vi "NEW数据采集传输系统.vi"() -> ()   [LabVIEW 2016, in "数据传输系统.lvlib"]
uses:
  <vilib>/Averna/Notify Icon/NotifyIcon.llb/BalloonIcon.ctl
  <vilib>/Utility/miscctls.llb/LVPointTypeDef.ctl
  <vilib>/Utility/config.llb/Read Key (String).vi
  <vilib>/Averna/Notify Icon/NotifyIcon.llb/GetSelectedItemEvent.vi
  <vilib>/Averna/Notify Icon/NotifyIcon.llb/SetVisible.vi
  <vilib>/Averna/Notify Icon/NotifyIcon.llb/SetMenuDefaultItem.vi
  <vilib>/Averna/Notify Icon/NotifyIcon.llb/SetTipText.vi
  <vilib>/Utility/config.llb/NI_LVConfig.lvlib
  data/FreeMem.dll
  <vilib>/Averna/Notify Icon/NotifyIcon.llb/NotifyIcon.lvclass
panel:
  out "错误输出":errorcluster
  in  "停止输入":bool caption="停止 2"
  in  "系统编码选择框":string(combo)="地表水质量监测"
  in  "数据发送通道":enum16{"TCP", "VISA"}(ring)
  in  "baud rate":u32=9600 caption="波特率"
  in  "VISA resource name":refnum<visa-resource-name> caption="VISA资源名称"
  in  "实时数据发送时间间隔/min":i32=1
  in  "数据组合发送":bool
  in  "日志、参数发送":bool
  in  "2011发送":bool
  in  "判断数据反馈":bool
  in  "数据发送协议":enum16{"2005-212协议", "2017-212协议"}(ring)=enum."2017-212协议"
  in  "重发时间":T1(ring)
  in  "重发日期":T2(ring)
  in  "开机启动":bool
  in  "确定更改起始时间":bool
  in  "更改起始时间":bool
  in  "数据发送起始时间":timestamp format="%<%.3X\n%Y/%m/%d>T"
  in  "每周自动重发":bool=TRUE
  in  "确定":bool
  in  "返回":bool
  in  "PW":string
  in  "MN":string
  in  "PORT":string
  in  "IP":string
  in  "站点设备":string
  in  "站点名称":string
  out "设置超时时间/min":i32=1
  out "状态信息":T3={"1st Error to Convert "=63, "步骤 "=enum."发送数据", "元素"="实时数据", "TCP服务端掉线计数"=0, "TCP掉线时间节点"="2019/05/08 15:24:17"} {"1st Error to Convert" items=["无错误", "参数错误", "内存已满", "超出区域", "文件结束", "文件已打开", "一般文件IO错误", "未找到文件", "文件权限错误", "磁盘已满", "路径副本", "打开过多文件", "未启用", "未找到资源文件", "无法添加资源", "未找到资源", "未找到图像", "图像内存错误", "画笔不存在", "配置错误类型", "配置未找到解析段", "配置解析错误", "配置内存错误", "错误外部代码格式", "错误外部代码偏移量", "外部代码不存在", "空窗口", "销毁窗口错误", "空菜单", "打印已中止", "错误打印记录", "打印驱动程序错误", "打印时窗口错误", "打印时内存错误", "打印对话框错误", "一般打印错误", "无效设备引用句柄", "设备未找到", "设备参数错误", "设备单位错误", "无法打开设备", "设备调用已中止", "一般错误", "用户已取消", "对象ID过低", "对象ID过高", "对象不在堆中", "未知的堆", "错误DefProc ID", "DefProc不在表格中", "范围外信息", "空方法", "未知信息", "不支持管理器调用", "错误地址", "连接过程中", "连接超时", "连接过程中", "不支持网络属性", "网络错误", "正在使用的地址", "系统缺少内存", "连接已中止", "连接已拒绝", "连接未建立", "连接已建立", "连接已关闭", "初始化错误（交互应用程序管理器）", "错误事件发生", "等待无约束事件发生处理程序", "事件发生队列溢出", "错误路径", "未发出信号量", "未识别类型（交互应用程序管理器）"]}
  out "数据接收超时指示灯":bool
  out "空闲时间/s":string
  out "系统时间":string
  out "实时小时数据上传":bool
  out "系统状态改变":bool
  out "软件版本":string
  out "掉线指示":bool
  out "核查数据上传":bool
  out "配置信息":T4
  in  "参数配置":bool
  out "反控数据发送":bool
  out "读取报文显示":string
  out "发送报文显示":string
  out "心跳包":bool
  out "通信状态":bool
  # "数 据 采 集 传 输 系 统"
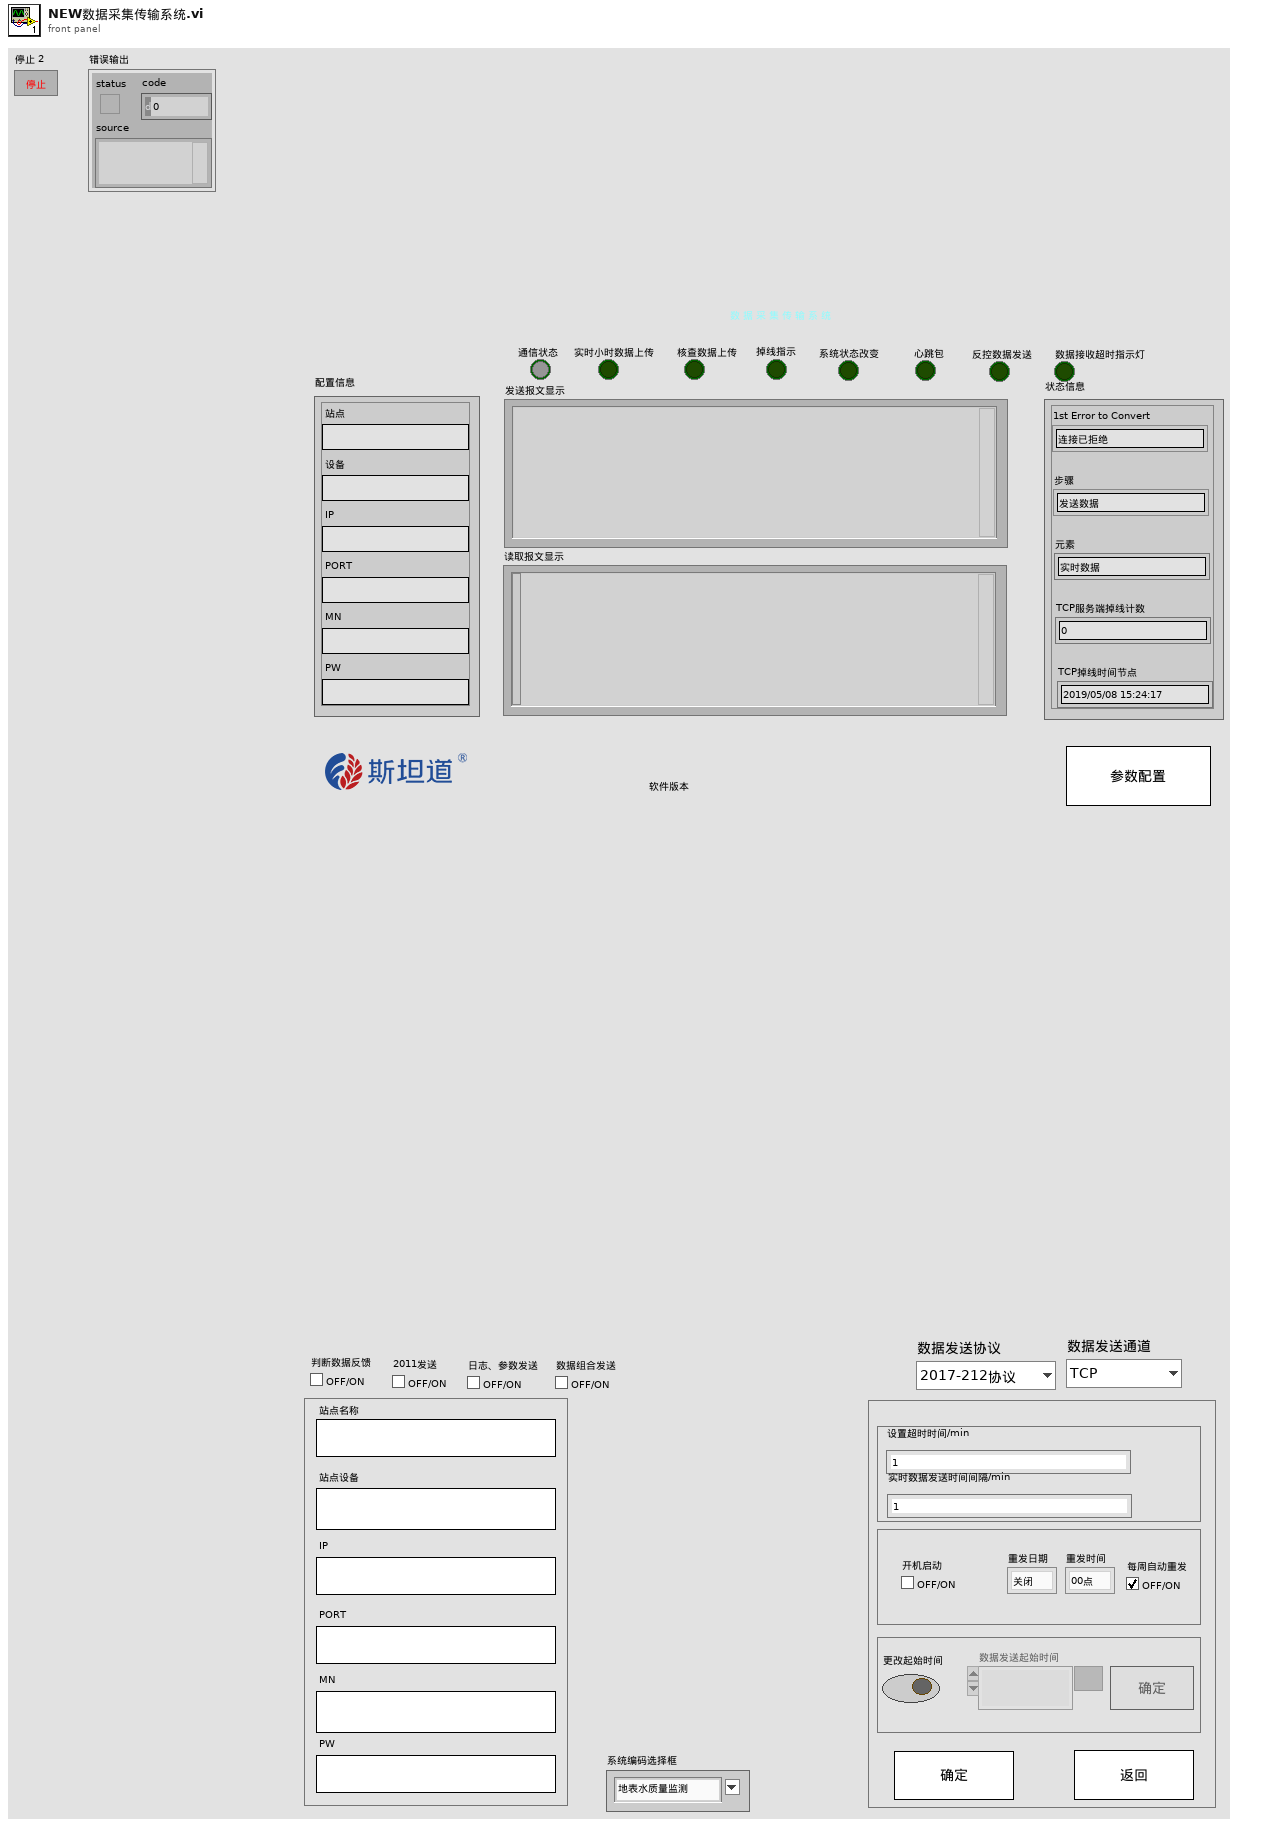
[diagram p1: front panel]
types:
  T1 = enum16{"00点", "01点", "02点", "03点", "04点", "05点", "06点", "07点", "08点", "09点", "10点", "11点", "12点", "13点", "14点", "15点", "16点", "17点", "18点", "19点", "20点", "21点", "22点", "23点"}
  T2 = enum16{"关闭", "星期日", "星期一", "星期二", "星期三", "星期四", "星期五", "星期六"}
  T3 = cluster{"1st Error to Convert ":i32, "步骤 ":enum16{"打开连接", "发送数据", "读取数据", "数据处理", "关闭连接"}, "元素":string, "TCP服务端掉线计数":i32, "TCP掉线时间节点":string}
  T4 = cluster{"站点":string, "设备":string, "IP":string, "PORT":string, "MN":string, "PW":string}
  T5 = typedef "LVPointTypeDef.ctl" = cluster{"Horizontal":i16, "Vertical":i16}
  T6 = cluster{"CODMn":bool, "CODCr":bool, "DO":bool, "铜":bool, "PH":bool, "氨氮":bool, "比电导率":bool, "水温":bool, "盐度(海水)":bool, "浊度":bool, "总氮":bool, "总磷":bool, "叶绿素a":bool, "藻密度":bool, "水位":bool, "流速":bool, "瞬时流量":bool, "累积流量":bool}
  T7 = typedef "NI_LVConfig.lvlib/Config Data RefNum.ctl" = refnum<k1>
  T8 = typedef "LVDateTimeRec.ctl" = cluster{"秒数的小数部分":dbl, "秒":i32, "分":i32, "时":i32, "日":i32, "月":i32, "年":i32, "天数（周）":i32, "天数（年）":i32, "DST":i32}
  T9 = typedef "imagedata.ctl" = cluster{"image type":i32, "image depth":i32, "image":u8[], "mask":u8[], "colors":u32[], "Rectangle":cluster{"left":i16, "top":i16, "right":i16, "bottom":i16}}
  T10 = enum8{"Enabled", "Disabled", "Disabled and Grayed Out"}
  T11 = enum32{"invalid app kind", "Development System", "Run Time System", "Student Edition", "Embedded LabVIEW", "Evaluation", "Custom"}
  T12 = enum32{"Invalid", "Standard", "Closed", "Hidden", "Minimized", "Maximized"}
  T13 = typedef "NotifyIcon.lvlib/NotifyIcon.lvclass/BalloonIcon.ctl" = enum32{"None", "Information", "Warning", "Error"}
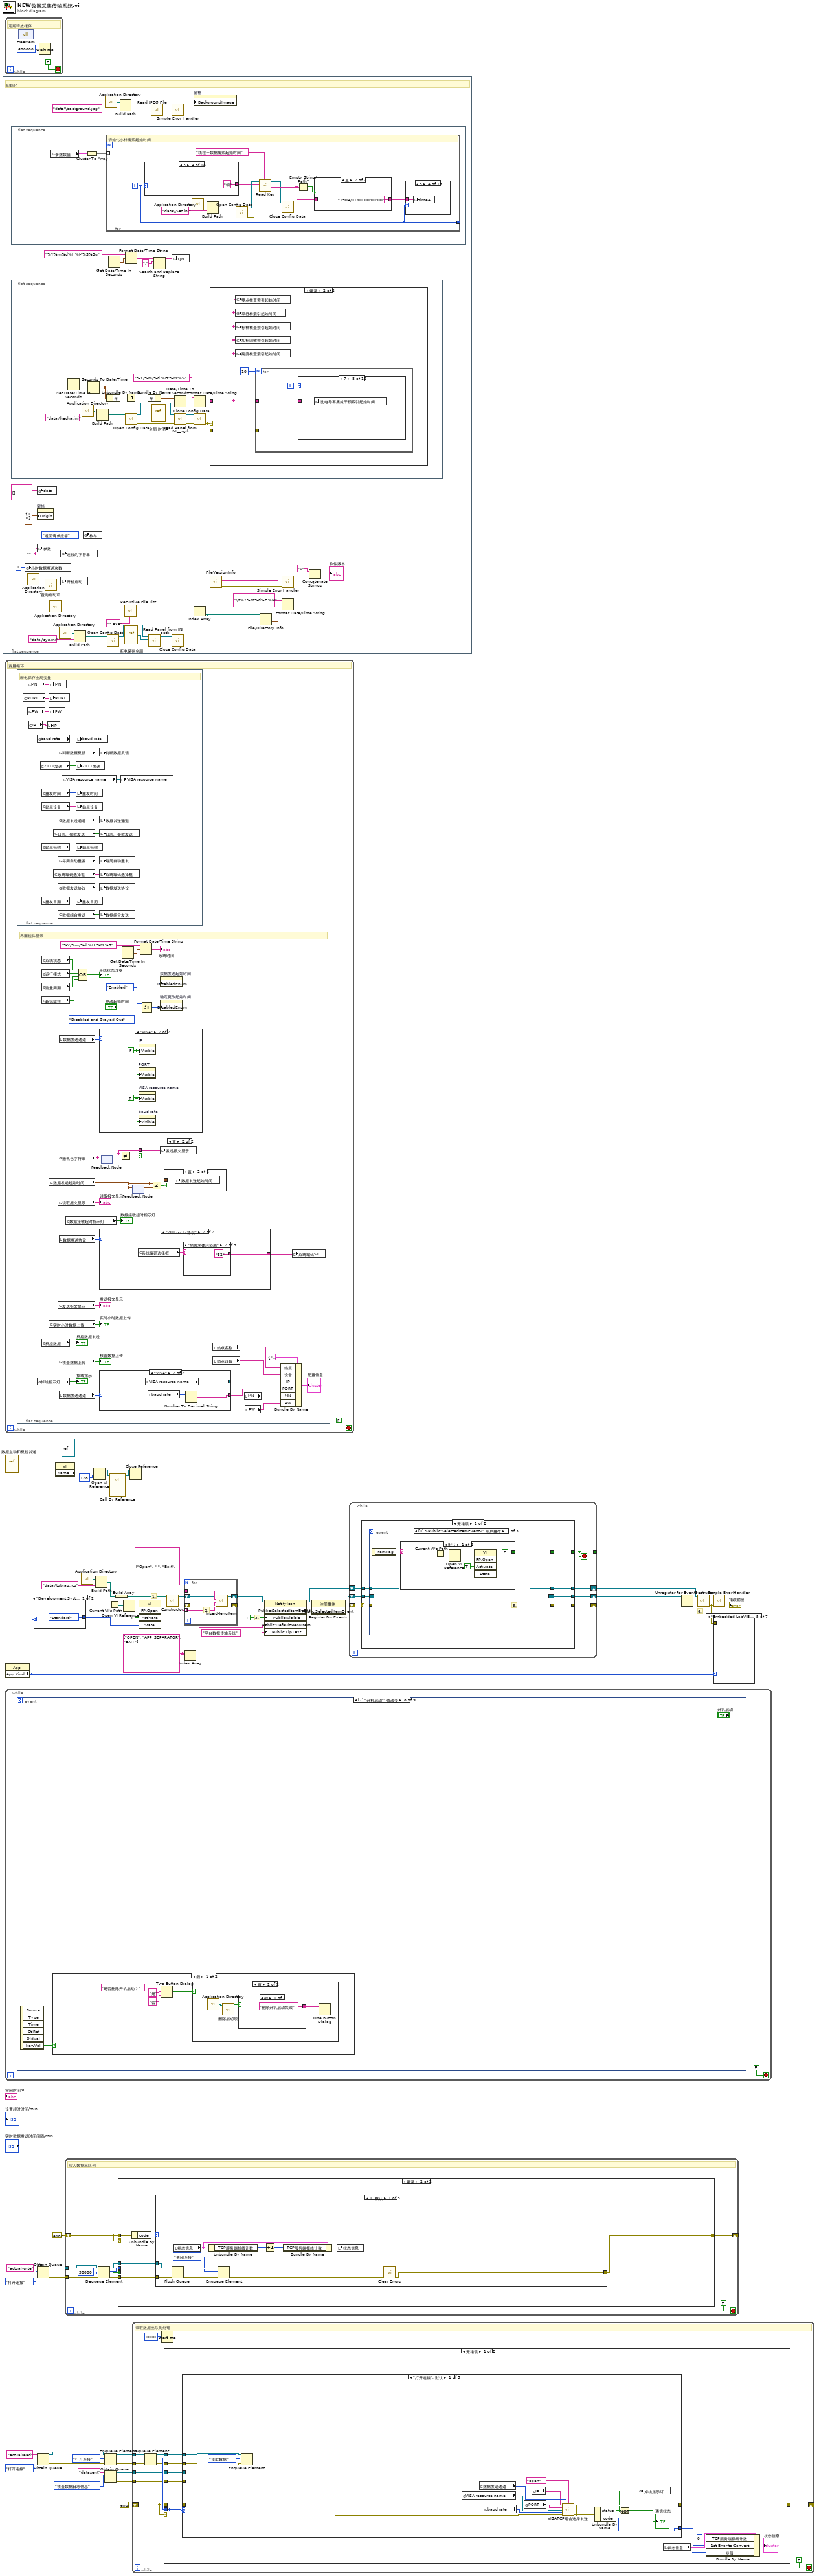
[diagram p0: block diagram]
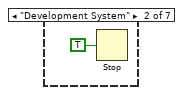
[diagram p3: hidden frame]
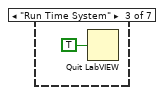
[diagram p4: hidden frame]
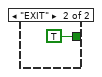
[diagram p8: hidden frame]
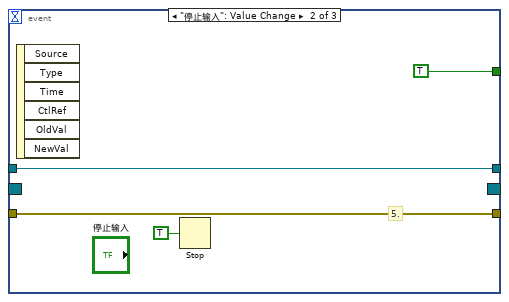
[diagram p9: hidden frame]
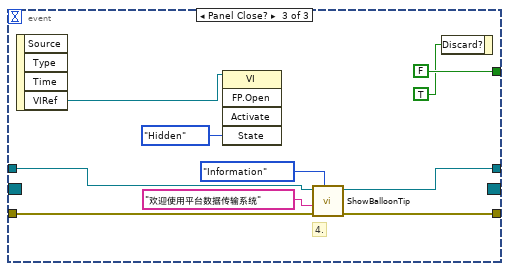
[diagram p10: hidden frame]
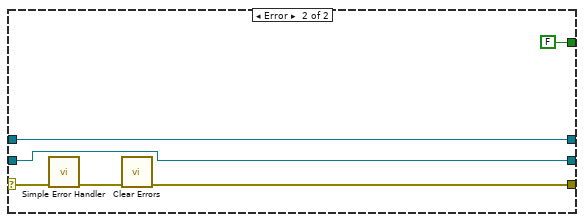
[diagram p11: hidden frame]
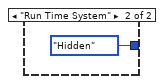
[diagram p12: hidden frame]
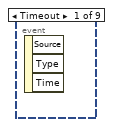
[diagram p13: hidden frame]
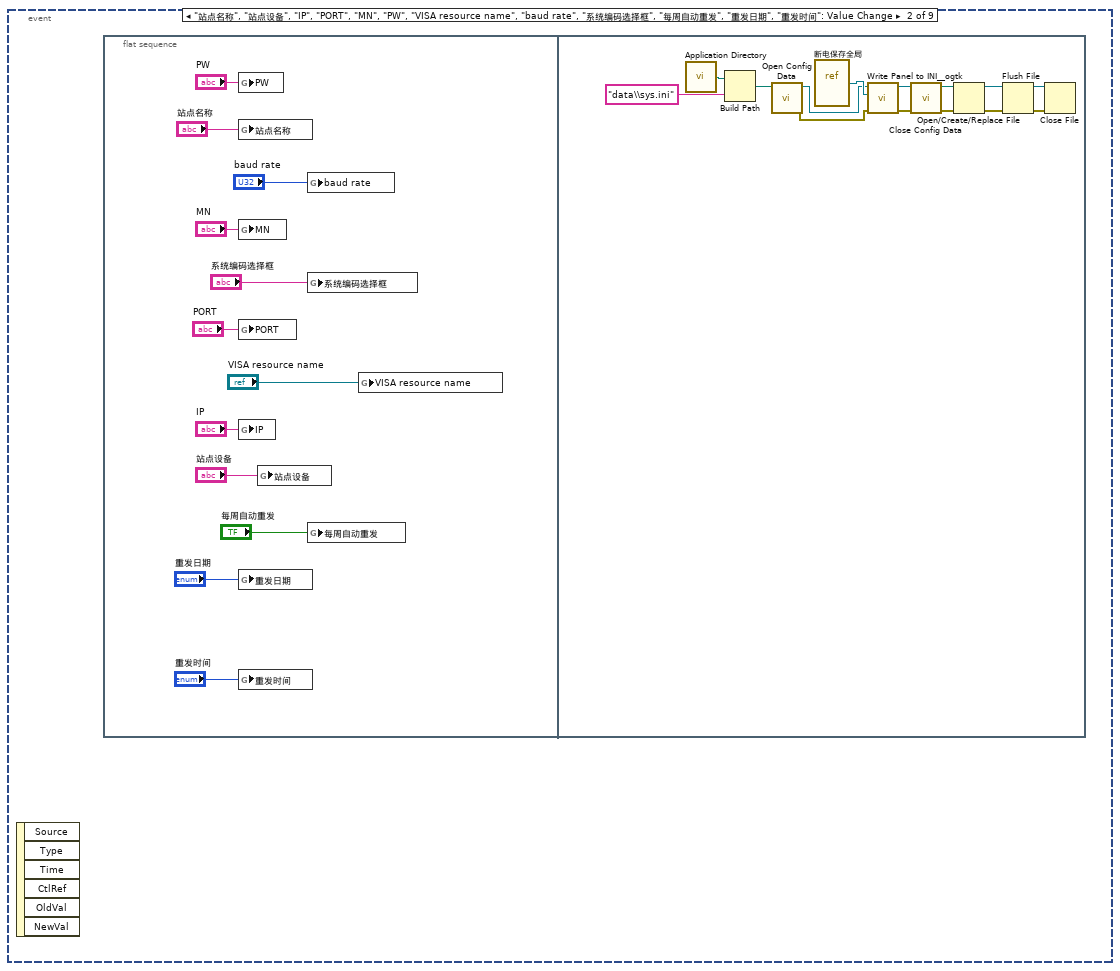
[diagram p14: hidden frame]
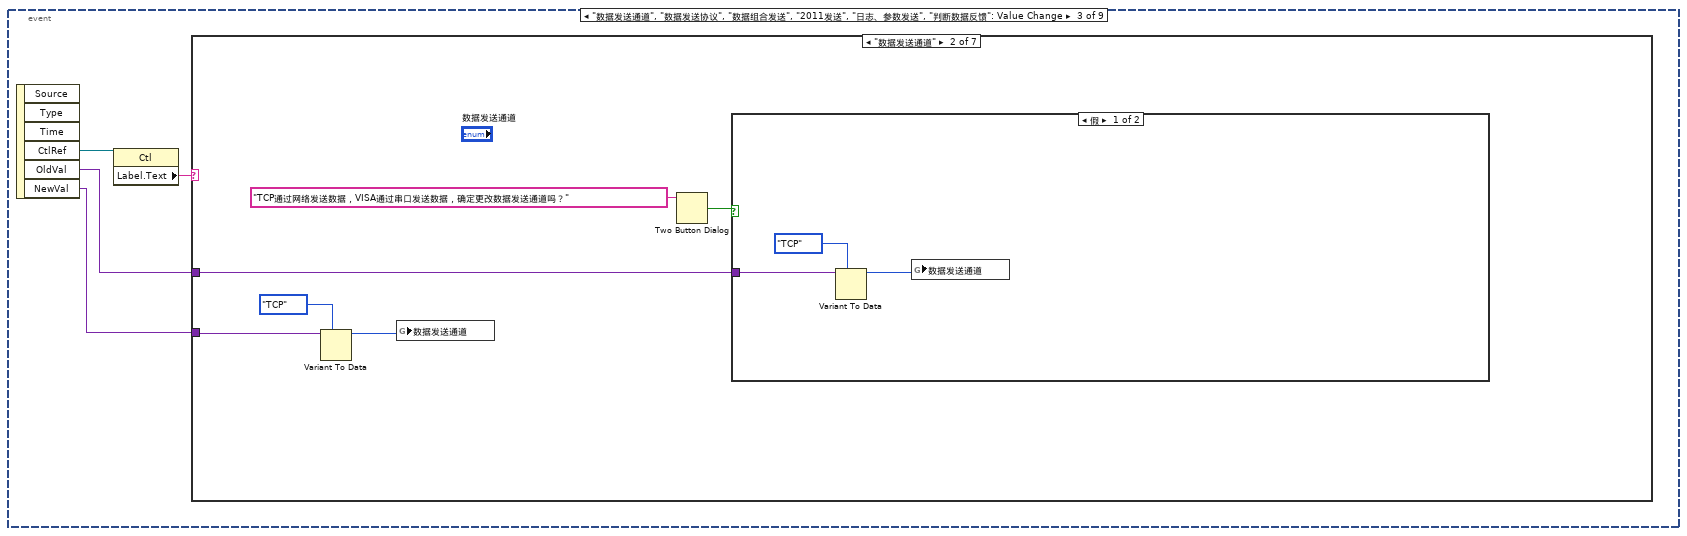
[diagram p15: hidden frame]
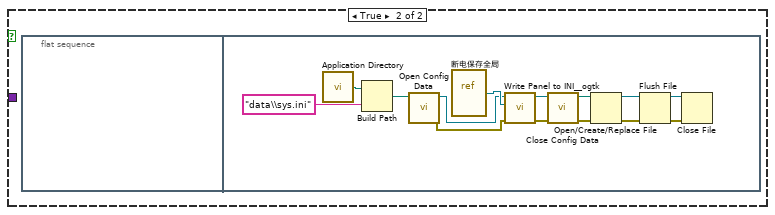
[diagram p17: hidden frame]
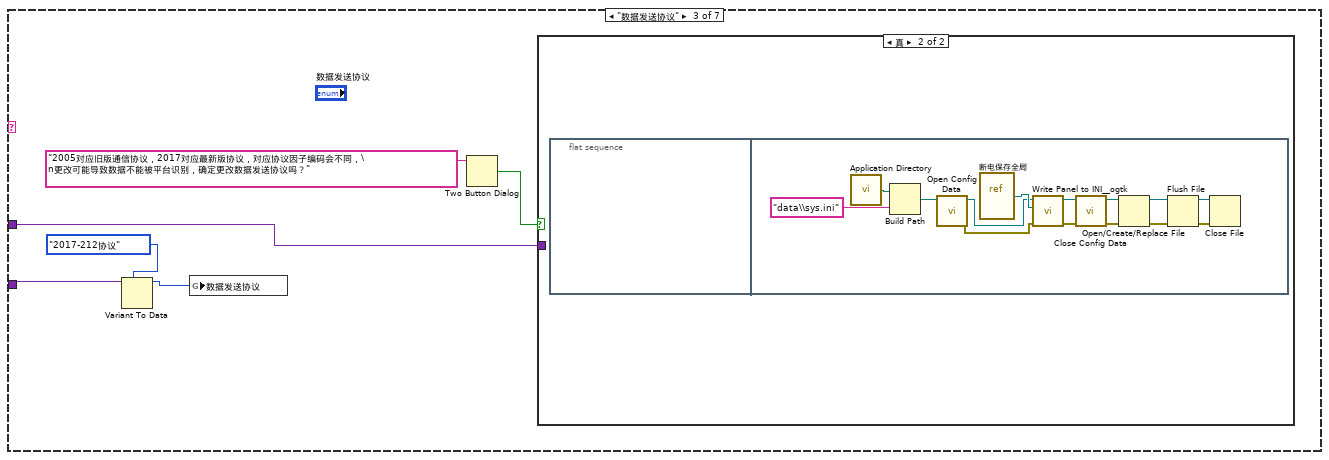
[diagram p18: hidden frame]
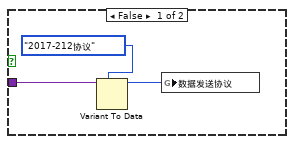
[diagram p19: hidden frame]
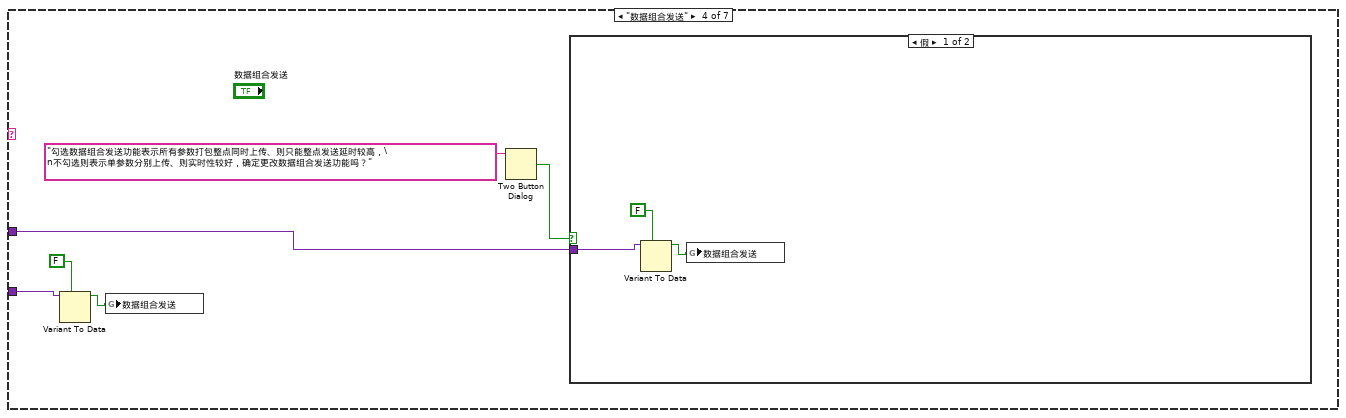
[diagram p20: hidden frame]
diagram:
  w13 = string[] ["OPEN", "APP_SEPARATOR", "EXIT"]
  # "6."
  # "3."
  # "1."
  n1 = flat-sequence {
    frame #0 {
      w89 = "" ("参数")
      # "初始化"
      n2 = flat-sequence {
        frame #0 {
          n3 = global read "全局1.vi" "参数数值"() -> (w92:T6)
          n4 = Cluster To Array(cluster=w92) -> (array=w93:bool[])
          n5 = for {
            tunnel: w93 -> [_] mode=indexing
            tunnel: [w96] -> _
            i -> [w96]
            # "初始化水样搜索起始时间"
            n6 = case shown="3" w96 {
              tunnel: ["CODMn" "CODCr" "DO" "铜" "PH" "氨氮" "比电导率" "水温" "盐度(海水)" "浊度" "总氮" "总磷" "叶绿素a" "藻密度" "水位" "流速" "瞬时流量" "累积流量"] -> w100
              frame 0, Default {
              }
              frame 1 {
              }
              frame 2 {
              }
              frame 3 {
              }
              frame 4 {
              }
              frame 5 {
              }
              frame 6 {
              }
              frame 7 {
              }
              frame 8 {
              }
              frame 9 {
              }
              frame 10 {
              }
              frame 11 {
              }
              frame 12 {
              }
              frame 13 {
              }
              frame 14 {
              }
              frame 15 {
              }
              frame 16 {
              }
              frame 17 {
              }
            }
            n7 = call <vilib>:"Application Directory.vi"() -> ("Application Directory"=w106:path)
            n8 = Build Path(base path=w106, name or relative path="data\\Set.ini" ("名称或相对路径")) -> (appended path=w104:path)
            n9 = call <vilib>:"Open Config Data.vi"("configuration file path"=w104) -> ("error out"=w102:errorcluster, "refnum"=w103:T7)  [unwired: 8 in, 1 out]
            n10 = call-poly <vilib>:"Read Key.vi"("section"="线程一数据搜索起始时间", "error in (no error)"=w102, "key"=w100, "refnum"=w103) -> ("error out"=w94:errorcluster, "value"=w97:string, "refnum out"=w95:T7)  [unwired: 4 in, 1 out]
            n11 = call <vilib>:"Close Config Data.vi"("error in (no error)"=w94, "refnum"=w95) -> ()  [unwired: 8 in, 2 out]
            n12 = Empty String/Path?(string/path=w97) -> (empty?=w99:bool)
            n13 = case shown="真" w99 {
              tunnel: [w107 "1904/01/01 00:00:00"] -> w98
              tunnel: w97 -> [w107 _]
              frame False {
              }
              frame True {
              }
            }
            n14 = case shown="3" w96 {
              tunnel: w98 -> [w109 w110 w111 w112 w113 w114 w115 w116 w117 w118 w119 w120 w121 w122 w123 w124 w125 w126]
              frame 0, Default {
                n15 = global write "全局 水样时间.vi" "time1"(w109) -> ()
              }
              frame 1 {
                n16 = global write "全局 水样时间.vi" "time2"(w110) -> ()
              }
              frame 2 {
                n17 = global write "全局 水样时间.vi" "time3"(w111) -> ()
              }
              frame 3 {
                n18 = global write "全局 水样时间.vi" "time4"(w112) -> ()
              }
              frame 4 {
                n19 = global write "全局 水样时间.vi" "time5"(w113) -> ()
              }
              frame 5 {
                n20 = global write "全局 水样时间.vi" "time6"(w114) -> ()
              }
              frame 6 {
                n21 = global write "全局 水样时间.vi" "time7"(w115) -> ()
              }
              frame 7 {
                n22 = global write "全局 水样时间.vi" "time8"(w116) -> ()
              }
              frame 8 {
                n23 = global write "全局 水样时间.vi" "time9"(w117) -> ()
              }
              frame 9 {
                n24 = global write "全局 水样时间.vi" "time10"(w118) -> ()
              }
              frame 10 {
                n25 = global write "全局 水样时间.vi" "time11"(w119) -> ()
              }
              frame 11 {
                n26 = global write "全局 水样时间.vi" "time12"(w120) -> ()
              }
              frame 12 {
                n27 = global write "全局 水样时间.vi" "time13"(w121) -> ()
              }
              frame 13 {
                n28 = global write "全局 水样时间.vi" "time14"(w122) -> ()
              }
              frame 14 {
                n29 = global write "全局 水样时间.vi" "time15"(w123) -> ()
              }
              frame 15 {
                n30 = global write "全局 水样时间.vi" "time16"(w124) -> ()
              }
              frame 16 {
                n31 = global write "全局 水样时间.vi" "time17"(w125) -> ()
              }
              frame 17 {
                n32 = global write "全局 水样时间.vi" "time18"(w126) -> ()
              }
            }
          }
        }
      }
      n33 = flat-sequence {
        frame #0 {
          n34 = Get Date/Time In Seconds() -> (seconds since 1Jan1904=w161:timestamp)
          n35 = call <vilib>:"Application Directory.vi"() -> ("Application Directory"=w151:path)
          n36 = Seconds To Date/Time(time stamp (now)=w161) -> (date time rec=w159:T8)  [unwired: 1 in]
          n37 = Build Path(base path=w151, name or relative path="data\\hecha.ini" ("名称或相对路径")) -> (appended path=w153:path)
          n38 = Unbundle By Name(w159) -> ("年"=w160:i32)
          n39 = Decrement(x=w160) -> (x-1=w158:i32)
          n40 = call <vilib>:"Open Config Data.vi"("configuration file path"=w153) -> ("error out"=w147:errorcluster, "refnum"=w148:T7)  [unwired: 8 in, 1 out]
          n41 = Bundle By Name(cluster=w159, "年"=w158) -> (w156:T8)
          n42 = vi-ref "全局 时间2.vi"() -> (w149:refnum<vi>)
          n43 = Date/Time To Seconds(2:w156) -> (0:w157:timestamp)  [unwired: 1 in]
          n44 = call <userlib>:"Read Panel from INI__ogtk.vi"("error in (no error)"=w147, "VI ref"=w149, "refnum"=w148) -> ("error out"=w146:errorcluster, "refnum out"=w150:T7)  [unwired: 7 in]
          n45 = Format Date/Time String(time format string (%c)="%Y/%m/%d %H:%M:%S" ("时间格式字符串(%c)"), seconds (now)=w157) -> (date/time string=w154:string)  [unwired: 1 in]
          n46 = call <vilib>:"Close Config Data.vi"("error in (no error)"=w146, "refnum"=w150) -> ("error out"=w145:errorcluster)  [unwired: 8 in, 1 out]
          n47 = case shown="错误" w145 {
            tunnel: w154 -> [_ w164]
            tunnel: w145 -> [_ w163]
            frame No Error {
            }
            frame Error {
              n48 = global write "全局 时间2.vi" "零点核查索引起始时间"(w164) -> ()
              n49 = global write "全局 时间2.vi" "平行样索引起始时间"(w164) -> ()
              n50 = global write "全局 时间2.vi" "标样核查索引起始时间"(w164) -> ()
              n51 = global write "全局 时间2.vi" "加标回收索引起始时间"(w164) -> ()
              n52 = global write "全局 时间2.vi" "跨度核查索引起始时间"(w164) -> ()
              n53 = for {
                N: 10 -> [_]
                tunnel: w164 -> [w165]
                tunnel: w163 -> [_]
                i -> [w166]
                n54 = case shown="7" w166 {
                  tunnel: w165 -> [w167 w168 w169 w170 w171 w172 w173 w174 w175 w176]
                  frame 0, Default {
                    n55 = global write "全局 时间2.vi" "氨氮平行样索引起始时间"(w167) -> ()
                    n56 = global write "全局 时间2.vi" "氨氮零点核查索引起始时间"(w167) -> ()
                    n57 = global write "全局 时间2.vi" "氨氮集成干预索引起始时间"(w167) -> ()
                    n58 = global write "全局 时间2.vi" "氨氮跨度核查索引起始时间"(w167) -> ()
                  }
                  frame 1 {
                    n59 = global write "全局 时间2.vi" "总氮零点核查索引起始时间"(w168) -> ()
                    n60 = global write "全局 时间2.vi" "总氮平行样索引起始时间"(w168) -> ()
                    n61 = global write "全局 时间2.vi" "总氮跨度核查索引起始时间"(w168) -> ()
                    n62 = global write "全局 时间2.vi" "总氮集成干预索引起始时间"(w168) -> ()
                  }
                  frame 2 {
                    n63 = global write "全局 时间2.vi" "总磷零点核查索引起始时间"(w169) -> ()
                    n64 = global write "全局 时间2.vi" "总磷平行样索引起始时间"(w169) -> ()
                    n65 = global write "全局 时间2.vi" "总磷跨度核查索引起始时间"(w169) -> ()
                    n66 = global write "全局 时间2.vi" "总磷集成干预索引起始时间"(w169) -> ()
                  }
                  frame 3 {
                    n67 = global write "全局 时间2.vi" "CODMn零点核查索引起始时间"(w170) -> ()
                    n68 = global write "全局 时间2.vi" "CODMn平行样索引起始时间"(w170) -> ()
                    n69 = global write "全局 时间2.vi" "CODMn跨度核查索引起始时间"(w170) -> ()
                    n70 = global write "全局 时间2.vi" "CODMn集成干预索引起始时间"(w170) -> ()
                  }
                  frame 4 {
                    n71 = global write "全局 时间2.vi" "CODCr零点核查索引起始时间"(w171) -> ()
                    n72 = global write "全局 时间2.vi" "CODCr平行样索引起始时间"(w171) -> ()
                    n73 = global write "全局 时间2.vi" "CODCr跨度核查索引起始时间"(w171) -> ()
                    n74 = global write "全局 时间2.vi" "CODCr集成干预索引起始时间"(w171) -> ()
                  }
                  frame 5 {
                    n75 = global write "全局 时间2.vi" "DO集成干预索引起始时间"(w172) -> ()
                  }
                  frame 6 {
                    n76 = global write "全局 时间2.vi" "PH集成干预索引起始时间"(w173) -> ()
                  }
                  frame 7 {
                    n77 = global write "全局 时间2.vi" "比电导率集成干预索引起始时间"(w174) -> ()
                  }
                  frame 8 {
                    n78 = global write "全局 时间2.vi" "水温集成干预索引起始时间"(w175) -> ()
                  }
                  frame 9 {
                    n79 = global write "全局 时间2.vi" "浊度集成干预索引起始时间"(w176) -> ()
                  }
                }
              }
            }
          }
        }
      }
      n80 = global write "全局 小时数据发送次数.vi" "小时数据发送次数"(0 ("数值")) -> ()
      n81 = call <vilib>:"Application Directory.vi"() -> ("Application Directory"=w57:path)
      n82 = global write "全局 实时数据参数.vi" "data"(string[][] [] ("data")) -> ()
      n83 = property on="窗格" class="Pane"("Origin"=T5 {"Horizontal"=0, "Vertical"=0} ("原点")) -> ()  [unwired: 2 in, 2 out]
      n84 = global write "全局 实时数据参数.vi" "参数"(w89) -> ()
      n85 = call "查询启动项.vi"("启动文件路径"=w57) -> ("包含启动项"=w56:bool)  [unwired: 9 in, 1 out]
      n86 = call <vilib>:"Application Directory.vi"() -> ("Application Directory"=w68:path)
      n87 = call <vilib>:"Application Directory.vi"() -> ("Application Directory"=w61:path)
      n88 = global write "全局 实时数据参数.vi" "连接的字符串"(w89) -> ()
      n89 = local write "开机启动"(w56) -> ()
      n90 = Build Path(base path=w61, name or relative path="data\\sys.ini" ("名称或相对路径")) -> (appended path=w59:path)
      n91 = global write "全局1.vi" "枚举"(enum16{"返回请求应答", "上传数据", "返回执行结果"}."返回请求应答" ("枚举")) -> ()
      n92 = call <vilib>:"Application Directory.vi"() -> ("Application Directory"=w80:path)
      n93 = call <vilib>:"Open Config Data.vi"("configuration file path"=w59) -> ("error out"=w65:errorcluster, "refnum"=w64:T7)  [unwired: 8 in, 1 out]
      n94 = Get Date/Time In Seconds() -> (seconds since 1Jan1904=w85:timestamp)
      n95 = Build Path(base path=w80, name or relative path="data\\background.jpg" ("名称或相对路径")) -> (appended path=w79:path)
      n96 = call <vilib>:"Recursive File List.vi"("pattern"="*.exe", "Folder Path"=w68) -> ("All Files in Dir"=w75:path[])  [unwired: 5 in, 4 out]
      n97 = vi-ref "断电保存全局.vi"() -> (w63:refnum<vi>)
      n98 = Format Date/Time String(time format string (%c)="%Y%m%d%H%M%S%3u" ("时间格式字符串(%c)"), seconds (now)=w85) -> (date/time string=w84:string)  [unwired: 1 in]
      n99 = call <userlib>:"Read Panel from INI__ogtk.vi"("error in (no error)"=w65, "VI ref"=w63, "refnum"=w64) -> ("error out"=w58:errorcluster, "refnum out"=w62:T7)  [unwired: 7 in]
      n100 = call <vilib>:"Read JPEG File.vi"("path to JPEG file"=w79) -> ("error out"=w77:errorcluster, "image data"=w78:T9)  [unwired: 8 in, 1 out]
      n101 = Search and Replace String(input string=w84, search string="." ("搜索字符串")) -> (result string=w82:string)  [unwired: 6 in, 3 out]
      n102 = call <vilib>:"Simple Error Handler.vi"("error in (no error)"=w77) -> ()  [unwired: 4 in, 5 out]
      n103 = global write "全局1.vi" "QN"(w82) -> ()
      n104 = call <vilib>:"Close Config Data.vi"("error in (no error)"=w58, "refnum"=w62) -> ()  [unwired: 8 in, 2 out]
      n105 = property on="窗格" class="Pane"("BackgroundImage"=w78) -> ()  [unwired: 2 in, 2 out]
      n106 = Index Array(array=w75) -> (element=w74:path)  [unwired: 1 in]
      n107 = call <vilib>:"FileVersionInfo.vi"("Application Path in"=w74) -> ("error out"=w67:errorcluster, "File Version Info"=w70:string)  [unwired: 7 in, 2 out]
      n108 = File/Directory Info(path=w74) -> (last mod=w73:timestamp)  [unwired: 1 in, 6 out]
      n109 = call <vilib>:"Simple Error Handler.vi"("error in (no error)"=w67) -> ()  [unwired: 4 in, 5 out]
      n110 = Format Date/Time String(time format string (%c)="\n%Y%m%d%H%M" ("时间格式字符串(%c)"), seconds (now)=w73) -> (date/time string=w69:string)  [unwired: 1 in]
      n111 = Concatenate Strings("V" ("字符串"), w70, w69) -> (→"软件版本":string)
    }
  }
  n112 = while {
    stop <- FALSE stop-if-true
    # "定期释放缓存"
    n113 = dll-call lib="PTH2aabs F\tgitkrakenCC6平台数采程序 - V2.0.1（正式修改迭代版）dataFreeMem.dll" fn="FreeMem"() -> ()  [unwired: 4 in, 2 out]
    n114 = Wait (ms)(milliseconds to wait=u32 600000 ("等待时间（毫秒）")) -> ()  [unwired: 1 out]
  }
  n115 = while {
    stop <- FALSE stop-if-true
    # "变量循环"
    n116 = flat-sequence {
      frame #0 {
        # "断电保存全局变量"
        n117 = global read "断电保存全局.vi" "PORT"() -> (w248:string)
        n118 = global read "断电保存全局.vi" "MN"() -> (w247:string)
        n119 = global read "断电保存全局.vi" "PW"() -> (w246:string)
        n120 = global read "断电保存全局.vi" "IP"() -> (w249:string)
        n121 = global read "断电保存全局.vi" "baud rate"() -> (w244:u32)
        n122 = global read "断电保存全局.vi" "2011发送"() -> (w240:bool)
        n123 = global read "断电保存全局.vi" "重发时间"() -> (w234:T1)
        n124 = global read "断电保存全局.vi" "站点设备"() -> (w250:string)
        n125 = global read "断电保存全局.vi" "站点名称"() -> (w251:string)
        n126 = global read "断电保存全局.vi" "重发日期"() -> (w242:T2)
        n127 = local write "IP"(w249) -> ()
        n128 = local write "MN"(w247) -> ()
        n129 = local write "PORT"(w248) -> ()
        n130 = local write "PW"(w246) -> ()
        n131 = global read "断电保存全局.vi" "日志、参数发送"() -> (w239:bool)
        n132 = global read "断电保存全局.vi" "系统编码选择框"() -> (w235:string)
        n133 = global read "断电保存全局.vi" "判断数据反馈"() -> (w241:bool)
        n134 = global read "断电保存全局.vi" "数据发送通道"() -> (w236:enum16{"TCP", "VISA"})
        n135 = global read "断电保存全局.vi" "每周自动重发"() -> (w243:bool)
        n136 = global read "断电保存全局.vi" "数据发送协议"() -> (w237:enum16{"2005-212协议", "2017-212协议"})
        n137 = global read "断电保存全局.vi" "数据组合发送"() -> (w238:bool)
        n138 = global read "断电保存全局.vi" "VISA resource name"() -> (w245:refnum<visa-resource-name>)
        n139 = local write "baud rate"(w244) -> ()
        n140 = local write "2011发送"(w240) -> ()
        n141 = local write "重发时间"(w234) -> ()
        n142 = local write "站点设备"(w250) -> ()
        n143 = local write "站点名称"(w251) -> ()
        n144 = local write "重发日期"(w242) -> ()
        n145 = local write "判断数据反馈"(w241) -> ()
        n146 = local write "数据发送通道"(w236) -> ()
        n147 = local write "日志、参数发送"(w239) -> ()
        n148 = local write "每周自动重发"(w243) -> ()
        n149 = local write "系统编码选择框"(w235) -> ()
        n150 = local write "数据发送协议"(w237) -> ()
        n151 = local write "数据组合发送"(w238) -> ()
        n152 = local write "VISA resource name"(w245) -> ()
      }
    }
    n153 = flat-sequence {
      frame #0 {
        # "界面控件显示"
        n154 = global read "全局 数据发送重叠.vi" "掉线指示灯"() -> (→"掉线指示":bool)
        n155 = global read "全局1.vi" "系统状态"() -> (w183:bool)
        n156 = global read "全局1.vi" "运行模式"() -> (w184:bool)
        n157 = global read "全局1.vi" "测量周期"() -> (w185:bool)
        n158 = global read "全局1.vi" "超标留样"() -> (w186:bool)
        n159 = global read "全局1.vi" "反控数据"() -> (→"反控数据发送":bool)
        n160 = global read "全局1.vi" "数据发送起始时间"() -> (w180:timestamp)
        n161 = global read "全局1.vi" "实时小时数据上传"() -> (→"实时小时数据上传":bool)
        n162 = global read "全局1.vi" "通讯包字符串"() -> (w197:string)
        n163 = global read "全局1.vi" "读取报文显示"() -> (→"读取报文显示":string)
        n164 = global read "全局1.vi" "发送报文显示"() -> (→"发送报文显示":string)
        n165 = global read "全局1.vi" "核查数据上传"() -> (→"核查数据上传":bool)
        n166 = local read "数据发送通道"() -> (w191:enum16{"TCP", "VISA"})
        n167 = local read "数据发送协议"() -> (w205:enum16{"2005-212协议", "2017-212协议"})
        n168 = local read "数据发送通道"() -> (w216:enum16{"TCP", "VISA"})
        n169 = global read "全局 数据发送重叠.vi" "数据接收超时指示灯"() -> (→"数据接收超时指示灯":bool)
        n170 = Compound Arithmetic op=OR ("复合运算")(w183, w184, w185, w186) -> (→"系统状态改变":bool)
        n171 = case shown="\"VISA\"" w191 {
          frame "TCP", Default {
            w218 = TRUE ("可见")
            w219 = FALSE ("可见")
            n172 = property on="IP" class="Str"("Visible"=w218) -> ()  [unwired: 2 in, 2 out]
            n173 = property on="PORT" class="Str"("Visible"=w218) -> ()  [unwired: 2 in, 2 out]
            n174 = property on="VISA resource name" class="VISAName"("Visible"=w219) -> ()  [unwired: 2 in, 2 out]
            n175 = property on="baud rate" class="DigNum (严格)"("Visible"=w219) -> ()  [unwired: 2 in, 2 out]
          }
          frame "VISA" {
            w220 = FALSE ("可见")
            w221 = TRUE ("可见")
            n176 = property on="IP" class="Str"("Visible"=w220) -> ()  [unwired: 2 in, 2 out]
            n177 = property on="PORT" class="Str"("Visible"=w220) -> ()  [unwired: 2 in, 2 out]
            n178 = property on="VISA resource name" class="VISAName"("Visible"=w221) -> ()  [unwired: 2 in, 2 out]
            n179 = property on="baud rate" class="DigNum (严格)"("Visible"=w221) -> ()  [unwired: 2 in, 2 out]
          }
        }
        n180 = case shown="\"2017-212协议\"" w205 {
          tunnel: ["32" ("设备编码MN") w224] -> w204
          frame "2005-212协议", Default {
          }
          frame "2017-212协议" {
            n181 = global read "断电保存全局.vi" "系统编码选择框"() -> (w225:string)
            n182 = case shown="\"地表水体污染源\"" w225 {
              tunnel: ["52" ("设备编码MN") "32" ("设备编码MN") "21" ("设备编码MN")] -> w224
              frame "污水排放过程监测" {
              }
              frame "地表水体污染源" {
              }
              frame "地表水质量监测", Default {
              }
            }
          }
        }
        n183 = case shown="\"VISA\"" w216 {
          tunnel: [w230 w233] -> w213
          tunnel: [w229 w231] -> w210
          frame "TCP", Default {
            n184 = local read "PORT"() -> (w229:string)
            n185 = local read "IP"() -> (w230:string)
          }
          frame "VISA" {
            n186 = local read "VISA resource name"() -> (w233:refnum<visa-resource-name>)
            n187 = local read "baud rate"() -> (w232:u32)
            n188 = Number To Decimal String(number=w232) -> (decimal integer string=w231:string)  [unwired: 1 in]
          }
        }
        n189 = feedback #1(w197) -> (w198:string)
        n190 = feedback-in #1(w197) -> ()
        n191 = Not Equal?(x=w197, y=w198) -> (x != y?=w196:bool)
        n192 = Get Date/Time In Seconds() -> (seconds since 1Jan1904=w206:timestamp)
        n193 = feedback #2(w180) -> (w182:timestamp)
        n194 = feedback-in #2(w180) -> ()
        n195 = case shown="真" w196 {
          tunnel: w197 -> [_ w222]
          frame False {
          }
          frame True {
            n196 = global write "全局1.vi" "发送报文显示"(w222) -> ()
          }
        }
        n197 = Format Date/Time String(time format string (%c)="%Y/%m/%d %H:%M:%S" ("时间格式字符串(%c)"), seconds (now)=w206) -> (date/time string=→"系统时间":string)  [unwired: 1 in]
        n198 = Select(t=T10."Enabled" ("禁用"), s="更改起始时间", f=T10."Disabled and Grayed Out" ("禁用")) -> (s? t:f=w192:T10)
        n199 = Not Equal?(x=w180, y=w182) -> (x != y?=w181:bool)
        n200 = property on="数据发送起始时间" class="AbsTime (严格)"("DisabledEnum"=w192) -> ()  [unwired: 2 in, 2 out]
        n201 = property on="确定更改起始时间" class="Bool"("DisabledEnum"=w192) -> ()  [unwired: 2 in, 2 out]
        n202 = case shown="真" w181 {
          tunnel: w180 -> [_ w217]
          frame False {
          }
          frame True {
            n203 = local write "数据发送起始时间"(w217) -> ()
          }
        }
        n204 = local read "站点名称"() -> (w212:string)
        n205 = local read "站点设备"() -> (w211:string)
        n206 = local read "MN"() -> (w209:string)
        n207 = local read "PW"() -> (w208:string)
        n208 = Bundle By Name(cluster=T4 {"站点"="", "设备"="", "IP"="", "PORT"="", "MN"="", "PW"=""} ("配置信息"), "站点"=w212, "设备"=w211, "IP"=w213, "PORT"=w210, "MN"=w209, "PW"=w208) -> (→"配置信息":T4)
        n209 = global write "全局1.vi" "系统编码ST"(w204) -> ()
      }
    }
  }
  n210 = vi-ref "数据主动和反控发送.vi"() -> (w42:refnum<vi>)
  n211 = property class="App"() -> ("App.Kind"=w5:T11)  [unwired: 2 in, 2 out]
  n212 = while {
    stop <- FALSE stop-if-true
    n213 = event shown="[7] \"开机启动\": 值改变" {
      selector: _ -> [_ _ _ _ _ _ _ _ _]
      dyn-events: _ -> [_ _ _ _ _ _ _ _ _]
      timeout: _ -> [_ _ _ _ _ _ _ _ _]
      event Timeout {
        n214 = event-data() -> ()  [unwired: 1 in, 3 out]
      }
      event "站点名称", "站点设备", "IP", "PORT", "MN", "PW", "VISA resource name", "baud rate", "系统编码选择框", "每周自动重发", "重发日期", "重发时间": Value Change {
        n215 = event-data() -> ()  [unwired: 1 in, 6 out]
        n216 = flat-sequence {
          frame #0 {
            n217 = global write "断电保存全局.vi" "PW"("PW") -> ()
            n218 = global write "断电保存全局.vi" "站点名称"("站点名称") -> ()
            n219 = global write "断电保存全局.vi" "MN"("MN") -> ()
            n220 = global write "断电保存全局.vi" "PORT"("PORT") -> ()
            n221 = global write "断电保存全局.vi" "IP"("IP") -> ()
            n222 = global write "断电保存全局.vi" "重发日期"("重发日期") -> ()
            n223 = global write "断电保存全局.vi" "重发时间"("重发时间") -> ()
            n224 = global write "断电保存全局.vi" "站点设备"("站点设备") -> ()
            n225 = global write "断电保存全局.vi" "baud rate"("baud rate") -> ()
            n226 = global write "断电保存全局.vi" "系统编码选择框"("系统编码选择框") -> ()
            n227 = global write "断电保存全局.vi" "每周自动重发"("每周自动重发") -> ()
            n228 = global write "断电保存全局.vi" "VISA resource name"("VISA resource name") -> ()
          }
          frame #1 {
            n229 = call <vilib>:"Application Directory.vi"() -> ("Application Directory"=w265:path)
            n230 = Build Path(base path=w265, name or relative path="data\\sys.ini" ("名称或相对路径")) -> (appended path=w267:path)
            n231 = call <vilib>:"Open Config Data.vi"("configuration file path"=w267) -> ("error out"=w271:errorcluster, "refnum"=w268:T7)  [unwired: 8 in, 1 out]
            n232 = vi-ref "断电保存全局.vi"() -> (w269:refnum<vi>)
            n233 = call <userlib>:"Write Panel to INI__ogtk.vi"("error in (no error)"=w271, "VI ref"=w269, "refnum"=w268) -> ("error out"=w272:errorcluster, "refnum out"=w270:T7)  [unwired: 7 in]
            n234 = call <vilib>:"Close Config Data.vi"("error in (no error)"=w272, "refnum"=w270) -> ("error out"=w277:errorcluster, "file path"=w278:path)  [unwired: 8 in]
            n235 = Open/Create/Replace File(file path (use dialog)=w278, error in=w277) -> (refnum out=w274:refnum<file>, error out=w273:errorcluster)  [unwired: 4 in, 1 out]
            n236 = Flush File(refnum=w274, error in=w273) -> (refnum out=w275:refnum<file>, error out=w276:errorcluster)
            n237 = Close File(refnum=w275, error in=w276) -> ()  [unwired: 2 out]
          }
        }
      }
      event "数据发送通道", "数据发送协议", "数据组合发送", "2011发送", "日志、参数发送", "判断数据反馈": Value Change {
        n238 = event-data() -> ("CtlRef"=w282:refnum<vi>, "OldVal"=w280:variant, "NewVal"=w279:variant)  [unwired: 1 in, 3 out]
        n239 = property class="Ctl"(reference=w282) -> ("Label.Text"=w281:string)  [unwired: 1 in, 2 out]
        n240 = case shown="\"数据发送通道\"" w281 {
          tunnel: w280 -> [_ w286 w309 w332 w355 w378 w401]
          tunnel: w279 -> [_ w283 w306 w329 w352 w375 w398]
          frame "假", Default {
          }
          frame "数据发送通道" {
            n241 = Variant To Data(type=enum16{"TCP", "VISA"}."TCP" ("数据发送通道"), Variant=w283) -> (data=w284:enum16{"TCP", "VISA"})  [unwired: 1 in, 1 out]
            n242 = global write "断电保存全局.vi" "数据发送通道"(w284) -> ()
            n243 = Two Button Dialog(message="TCP通过网络发送数据，VISA通过串口发送数据，确定更改数据发送通道吗？" ("消息")) -> (T button?=w287:bool)  [unwired: 2 in]
            n244 = case shown="假" w287 {
              tunnel: w286 -> [w290 _]
              frame False {
                n245 = Variant To Data(type=enum16{"TCP", "VISA"}."TCP" ("数据发送通道"), Variant=w290) -> (data=w289:enum16{"TCP", "VISA"})  [unwired: 1 in, 1 out]
                n246 = global write "断电保存全局.vi" "数据发送通道"(w289) -> ()
              }
              frame True {
                n247 = flat-sequence {
                  frame #0 {
                  }
                  frame #1 {
                    n248 = call <vilib>:"Application Directory.vi"() -> ("Application Directory"=w292:path)
                    n249 = Build Path(base path=w292, name or relative path="data\\sys.ini" ("名称或相对路径")) -> (appended path=w294:path)
                    n250 = call <vilib>:"Open Config Data.vi"("configuration file path"=w294) -> ("error out"=w298:errorcluster, "refnum"=w295:T7)  [unwired: 8 in, 1 out]
                    n251 = vi-ref "断电保存全局.vi"() -> (w296:refnum<vi>)
                    n252 = call <userlib>:"Write Panel to INI__ogtk.vi"("error in (no error)"=w298, "VI ref"=w296, "refnum"=w295) -> ("error out"=w299:errorcluster, "refnum out"=w297:T7)  [unwired: 7 in]
                    n253 = call <vilib>:"Close Config Data.vi"("error in (no error)"=w299, "refnum"=w297) -> ("error out"=w304:errorcluster, "file path"=w305:path)  [unwired: 8 in]
                    n254 = Open/Create/Replace File(file path (use dialog)=w305, error in=w304) -> (refnum out=w301:refnum<file>, error out=w300:errorcluster)  [unwired: 4 in, 1 out]
                    n255 = Flush File(refnum=w301, error in=w300) -> (refnum out=w302:refnum<file>, error out=w303:errorcluster)
                    n256 = Close File(refnum=w302, error in=w303) -> ()  [unwired: 2 out]
                  }
                }
              }
            }
          }
          frame "数据发送协议" {
            n257 = Variant To Data(type=enum16{"2005-212协议", "2017-212协议"}."2017-212协议" ("数据"), Variant=w306) -> (data=w307:enum16{"2005-212协议", "2017-212协议"})  [unwired: 1 in, 1 out]
            n258 = global write "断电保存全局.vi" "数据发送协议"(w307) -> ()
            n259 = Two Button Dialog(message="2005对应旧版通信协议，2017对应最新版协议，对应协议因子编码会不同，\n更改可能导致数据不能被平台识别，确定更改数据发送协议吗？" ("消息")) -> (T button?=w310:bool)  [unwired: 2 in]
            n260 = case shown="真" w310 {
              tunnel: w309 -> [w314 _]
              frame False {
                n261 = Variant To Data(type=enum16{"2005-212协议", "2017-212协议"}."2017-212协议" ("数据"), Variant=w314) -> (data=w312:enum16{"2005-212协议", "2017-212协议"})  [unwired: 1 in, 1 out]
                n262 = global write "断电保存全局.vi" "数据发送协议"(w312) -> ()
              }
              frame True {
                n263 = flat-sequence {
                  frame #0 {
                  }
                  frame #1 {
                    n264 = call <vilib>:"Application Directory.vi"() -> ("Application Directory"=w315:path)
                    n265 = Build Path(base path=w315, name or relative path="data\\sys.ini" ("名称或相对路径")) -> (appended path=w317:path)
                    n266 = call <vilib>:"Open Config Data.vi"("configuration file path"=w317) -> ("error out"=w321:errorcluster, "refnum"=w318:T7)  [unwired: 8 in, 1 out]
                    n267 = vi-ref "断电保存全局.vi"() -> (w319:refnum<vi>)
                    n268 = call <userlib>:"Write Panel to INI__ogtk.vi"("error in (no error)"=w321, "VI ref"=w319, "refnum"=w318) -> ("error out"=w322:errorcluster, "refnum out"=w320:T7)  [unwired: 7 in]
                    n269 = call <vilib>:"Close Config Data.vi"("error in (no error)"=w322, "refnum"=w320) -> ("error out"=w327:errorcluster, "file path"=w328:path)  [unwired: 8 in]
                    n270 = Open/Create/Replace File(file path (use dialog)=w328, error in=w327) -> (refnum out=w324:refnum<file>, error out=w323:errorcluster)  [unwired: 4 in, 1 out]
                    n271 = Flush File(refnum=w324, error in=w323) -> (refnum out=w325:refnum<file>, error out=w326:errorcluster)
                    n272 = Close File(refnum=w325, error in=w326) -> ()  [unwired: 2 out]
                  }
                }
              }
            }
          }
          frame "数据组合发送" {
            n273 = Variant To Data(type=FALSE, Variant=w329) -> (data=w330:bool)  [unwired: 1 in, 1 out]
            n274 = global write "断电保存全局.vi" "数据组合发送"(w330) -> ()
            n275 = Two Button Dialog(message="勾选数据组合发送功能表示所有参数打包整点同时上传、则只能整点发送延时较高，\n不勾选则表示单参数分别上传、则实时性较好，确定更改数据组合发送功能吗？" ("消息")) -> (T button?=w333:bool)  [unwired: 2 in]
            n276 = case shown="假" w333 {
              tunnel: w332 -> [w336 _]
              frame False {
                n277 = Variant To Data(type=FALSE, Variant=w336) -> (data=w335:bool)  [unwired: 1 in, 1 out]
                n278 = global write "断电保存全局.vi" "数据组合发送"(w335) -> ()
              }
              frame True {
                n279 = flat-sequence {
                  frame #0 {
                  }
                  frame #1 {
                    n280 = call <vilib>:"Application Directory.vi"() -> ("Application Directory"=w338:path)
                    n281 = Build Path(base path=w338, name or relative path="data\\sys.ini" ("名称或相对路径")) -> (appended path=w340:path)
                    n282 = call <vilib>:"Open Config Data.vi"("configuration file path"=w340) -> ("error out"=w344:errorcluster, "refnum"=w341:T7)  [unwired: 8 in, 1 out]
                    n283 = vi-ref "断电保存全局.vi"() -> (w342:refnum<vi>)
                    n284 = call <userlib>:"Write Panel to INI__ogtk.vi"("error in (no error)"=w344, "VI ref"=w342, "refnum"=w341) -> ("error out"=w345:errorcluster, "refnum out"=w343:T7)  [unwired: 7 in]
                    n285 = call <vilib>:"Close Config Data.vi"("error in (no error)"=w345, "refnum"=w343) -> ("error out"=w350:errorcluster, "file path"=w351:path)  [unwired: 8 in]
                    n286 = Open/Create/Replace File(file path (use dialog)=w351, error in=w350) -> (refnum out=w347:refnum<file>, error out=w346:errorcluster)  [unwired: 4 in, 1 out]
                    n287 = Flush File(refnum=w347, error in=w346) -> (refnum out=w348:refnum<file>, error out=w349:errorcluster)
                    n288 = Close File(refnum=w348, error in=w349) -> ()  [unwired: 2 out]
                  }
                }
              }
            }
          }
          frame "2011发送" {
            n289 = Variant To Data(type=FALSE, Variant=w352) -> (data=w353:bool)  [unwired: 1 in, 1 out]
            n290 = global write "断电保存全局.vi" "2011发送"(w353) -> ()
            n291 = Two Button Dialog(message="2011表示实时数据上传，一般情况需要勾选，确定更改2011实时数据发送功能吗？" ("消息")) -> (T button?=w356:bool)  [unwired: 2 in]
            n292 = case shown="真" w356 {
              tunnel: w355 -> [w359 _]
              frame False {
                n293 = Variant To Data(type=FALSE, Variant=w359) -> (data=w358:bool)  [unwired: 1 in, 1 out]
                n294 = global write "断电保存全局.vi" "2011发送"(w358) -> ()
              }
              frame True {
                n295 = flat-sequence {
                  frame #0 {
                  }
                  frame #1 {
                    n296 = call <vilib>:"Application Directory.vi"() -> ("Application Directory"=w361:path)
                    n297 = Build Path(base path=w361, name or relative path="data\\sys.ini" ("名称或相对路径")) -> (appended path=w363:path)
                    n298 = call <vilib>:"Open Config Data.vi"("configuration file path"=w363) -> ("error out"=w367:errorcluster, "refnum"=w364:T7)  [unwired: 8 in, 1 out]
                    n299 = vi-ref "断电保存全局.vi"() -> (w365:refnum<vi>)
                    n300 = call <userlib>:"Write Panel to INI__ogtk.vi"("error in (no error)"=w367, "VI ref"=w365, "refnum"=w364) -> ("error out"=w368:errorcluster, "refnum out"=w366:T7)  [unwired: 7 in]
                    n301 = call <vilib>:"Close Config Data.vi"("error in (no error)"=w368, "refnum"=w366) -> ("error out"=w373:errorcluster, "file path"=w374:path)  [unwired: 8 in]
                    n302 = Open/Create/Replace File(file path (use dialog)=w374, error in=w373) -> (refnum out=w370:refnum<file>, error out=w369:errorcluster)  [unwired: 4 in, 1 out]
                    n303 = Flush File(refnum=w370, error in=w369) -> (refnum out=w371:refnum<file>, error out=w372:errorcluster)
                    n304 = Close File(refnum=w371, error in=w372) -> ()  [unwired: 2 out]
                  }
                }
              }
            }
          }
          frame "日志、参数发送" {
            n305 = Variant To Data(type=FALSE, Variant=w375) -> (data=w376:bool)  [unwired: 1 in, 1 out]
            n306 = global write "断电保存全局.vi" "日志、参数发送"(w376) -> ()
            n307 = Two Button Dialog(message="选择是否需要仪器日志、状态和告警信息上传，一般情况需要勾选，确定更改日志、参数发送功能吗？" ("消息")) -> (T button?=w379:bool)  [unwired: 2 in]
            n308 = case shown="真" w379 {
              tunnel: w378 -> [w382 _]
              frame False {
                n309 = Variant To Data(type=FALSE, Variant=w382) -> (data=w381:bool)  [unwired: 1 in, 1 out]
                n310 = global write "断电保存全局.vi" "日志、参数发送"(w381) -> ()
              }
              frame True {
                n311 = flat-sequence {
                  frame #0 {
                  }
                  frame #1 {
                    n312 = call <vilib>:"Application Directory.vi"() -> ("Application Directory"=w384:path)
                    n313 = Build Path(base path=w384, name or relative path="data\\sys.ini" ("名称或相对路径")) -> (appended path=w386:path)
                    n314 = call <vilib>:"Open Config Data.vi"("configuration file path"=w386) -> ("error out"=w390:errorcluster, "refnum"=w387:T7)  [unwired: 8 in, 1 out]
                    n315 = vi-ref "断电保存全局.vi"() -> (w388:refnum<vi>)
                    n316 = call <userlib>:"Write Panel to INI__ogtk.vi"("error in (no error)"=w390, "VI ref"=w388, "refnum"=w387) -> ("error out"=w391:errorcluster, "refnum out"=w389:T7)  [unwired: 7 in]
                    n317 = call <vilib>:"Close Config Data.vi"("error in (no error)"=w391, "refnum"=w389) -> ("error out"=w396:errorcluster, "file path"=w397:path)  [unwired: 8 in]
                    n318 = Open/Create/Replace File(file path (use dialog)=w397, error in=w396) -> (refnum out=w393:refnum<file>, error out=w392:errorcluster)  [unwired: 4 in, 1 out]
                    n319 = Flush File(refnum=w393, error in=w392) -> (refnum out=w394:refnum<file>, error out=w395:errorcluster)
                    n320 = Close File(refnum=w394, error in=w395) -> ()  [unwired: 2 out]
                  }
                }
              }
            }
          }
          frame "判断数据反馈" {
            n321 = Variant To Data(type=FALSE, Variant=w398) -> (data=w399:bool)  [unwired: 1 in, 1 out]
            n322 = global write "断电保存全局.vi" "判断数据反馈"(w399) -> ()
            n323 = Two Button Dialog(message="勾选判断数据反馈是针对平台能有反馈的情况、此功能能保证数据的完整性，尽可能的防止各种问题导致的数据缺失，\n不勾选则表示数据只发送不判断平台的反馈、用于针对平台没有反馈的情况，确定更改判断数据反馈功能吗？" ("消息")) -> (T button?=w402:bool)  [unwired: 2 in]
            n324 = case shown="真" w402 {
              tunnel: w401 -> [w405 _]
              frame False {
                n325 = Variant To Data(type=FALSE, Variant=w405) -> (data=w404:bool)  [unwired: 1 in, 1 out]
                n326 = global write "断电保存全局.vi" "判断数据反馈"(w404) -> ()
              }
              frame True {
                n327 = flat-sequence {
                  frame #0 {
                  }
                  frame #1 {
                    n328 = call <vilib>:"Application Directory.vi"() -> ("Application Directory"=w407:path)
                    n329 = Build Path(base path=w407, name or relative path="data\\sys.ini" ("名称或相对路径")) -> (appended path=w409:path)
                    n330 = call <vilib>:"Open Config Data.vi"("configuration file path"=w409) -> ("error out"=w413:errorcluster, "refnum"=w410:T7)  [unwired: 8 in, 1 out]
                    n331 = vi-ref "断电保存全局.vi"() -> (w411:refnum<vi>)
                    n332 = call <userlib>:"Write Panel to INI__ogtk.vi"("error in (no error)"=w413, "VI ref"=w411, "refnum"=w410) -> ("error out"=w414:errorcluster, "refnum out"=w412:T7)  [unwired: 7 in]
                    n333 = call <vilib>:"Close Config Data.vi"("error in (no error)"=w414, "refnum"=w412) -> ("error out"=w419:errorcluster, "file path"=w420:path)  [unwired: 8 in]
                    n334 = Open/Create/Replace File(file path (use dialog)=w420, error in=w419) -> (refnum out=w416:refnum<file>, error out=w415:errorcluster)  [unwired: 4 in, 1 out]
                    n335 = Flush File(refnum=w416, error in=w415) -> (refnum out=w417:refnum<file>, error out=w418:errorcluster)
                    n336 = Close File(refnum=w417, error in=w418) -> ()  [unwired: 2 out]
                  }
                }
              }
            }
          }
        }
      }
      event "确定": Value Change {
        n337 = event-data() -> ()  [unwired: 1 in, 6 out]
        n338 = call "通信状态入队列.vi"("枚举"=enum16{"打开连接", "发送数据", "读取数据", "数据处理", "关闭连接"}."关闭连接") -> ()  [unwired: 10 in, 1 out]
      }
      event "参数配置": Value Change {
        n339 = event-data() -> ()  [unwired: 1 in, 6 out]
        n340 = property on="窗格" class="Pane"("Origin"=T5 {"Horizontal"=0, "Vertical"=1000} ("原点")) -> ()  [unwired: 2 in, 2 out]
      }
      event "返回": Value Change {
        n341 = event-data() -> ()  [unwired: 1 in, 6 out]
        n342 = property on="窗格" class="Pane"("Origin"=T5 {"Horizontal"=0, "Vertical"=0} ("原点")) -> ()  [unwired: 2 in, 2 out]
      }
      event "确定更改起始时间": Value Change {
        n343 = event-data() -> ()  [unwired: 1 in, 6 out]
        n344 = local write "更改起始时间"(FALSE ("更改起始时间")) -> ()
        n345 = Two Button Dialog(message="确定以当前设置时间作为数据索引起始时间？" ("消息")) -> (T button?=w424:bool)  [unwired: 2 in]
        n346 = case shown="真" w424 {
          frame False {
          }
          frame True {
            n347 = global read "全局1.vi" "参数数值"() -> (w427:T6)
            n348 = global write "断电保存全局.vi" "数据重发"(TRUE ("数据重发")) -> ()
            n349 = Cluster To Array(cluster=w427) -> (array=w431:bool[])
            n350 = for {
              tunnel: w431 -> [_] mode=indexing
              tunnel: [w442] -> w430
              i -> [w443]
              n351 = Format Date/Time String(time format string (%c)="%Y/%m/%d %H:%M:%S" ("时间格式字符串(%c)"), seconds (now)="数据发送起始时间") -> (date/time string=w442:string)  [unwired: 1 in]
              n352 = global write "断电保存全局.vi" "数据重发时间戳"(w442) -> ()
              n353 = case shown="0, 默认" w443 {
                tunnel: w442 -> [w445 w446 w447 w448 w449 w450 w451 w452 w453 w454 w455 w456 w457 w458 w459 w460 w461 w462]
                frame 0, Default {
                  n354 = global write "全局 水样时间.vi" "time1"(w445) -> ()
                }
                frame 1 {
                  n355 = global write "全局 水样时间.vi" "time2"(w446) -> ()
                }
                frame 2 {
                  n356 = global write "全局 水样时间.vi" "time3"(w447) -> ()
                }
                frame 3 {
                  n357 = global write "全局 水样时间.vi" "time4"(w448) -> ()
                }
                frame 4 {
                  n358 = global write "全局 水样时间.vi" "time5"(w449) -> ()
                }
                frame 5 {
                  n359 = global write "全局 水样时间.vi" "time6"(w450) -> ()
                }
                frame 6 {
                  n360 = global write "全局 水样时间.vi" "time7"(w451) -> ()
                }
                frame 7 {
                  n361 = global write "全局 水样时间.vi" "time8"(w452) -> ()
                }
                frame 8 {
                  n362 = global write "全局 水样时间.vi" "time9"(w453) -> ()
                }
                frame 9 {
                  n363 = global write "全局 水样时间.vi" "time10"(w454) -> ()
                }
                frame 10 {
                  n364 = global write "全局 水样时间.vi" "time11"(w455) -> ()
                }
                frame 11 {
                  n365 = global write "全局 水样时间.vi" "time12"(w456) -> ()
                }
                frame 12 {
                  n366 = global write "全局 水样时间.vi" "time13"(w457) -> ()
                }
                frame 13 {
                  n367 = global write "全局 水样时间.vi" "time14"(w458) -> ()
                }
                frame 14 {
                  n368 = global write "全局 水样时间.vi" "time15"(w459) -> ()
                }
                frame 15 {
                  n369 = global write "全局 水样时间.vi" "time16"(w460) -> ()
                }
                frame 16 {
                  n370 = global write "全局 水样时间.vi" "time17"(w461) -> ()
                }
                frame 17 {
                  n371 = global write "全局 水样时间.vi" "time18"(w462) -> ()
                }
              }
            }
            n372 = global read "断电保存全局.vi" "数据组合发送"() -> (w428:bool)
            n373 = case shown="假" w428 {
              tunnel: w430 -> [w432 _]
              frame False {
                n374 = global write "全局 时间2.vi" "标样核查索引起始时间"(w432) -> ()
                n375 = global write "全局 时间2.vi" "加标回收索引起始时间"(w432) -> ()
                n376 = global write "全局 时间2.vi" "跨度核查索引起始时间"(w432) -> ()
                n377 = global write "全局 时间2.vi" "零点核查索引起始时间"(w432) -> ()
                n378 = for {
                  N: 5 -> [_]
                  tunnel: w432 -> [w434]
                  i -> [w435]
                  n379 = case shown="1" w435 {
                    tunnel: w434 -> [w436 w437 w438 w439 w440]
                    frame 0, Default {
                      n380 = global write "全局 时间2.vi" "氨氮零点核查索引起始时间"(w436) -> ()
                      n381 = global write "全局 时间2.vi" "氨氮跨度核查索引起始时间"(w436) -> ()
                    }
                    frame 1 {
                      n382 = global write "全局 时间2.vi" "总氮零点核查索引起始时间"(w437) -> ()
                      n383 = global write "全局 时间2.vi" "总氮跨度核查索引起始时间"(w437) -> ()
                    }
                    frame 2 {
                      n384 = global write "全局 时间2.vi" "总磷零点核查索引起始时间"(w438) -> ()
                      n385 = global write "全局 时间2.vi" "总磷跨度核查索引起始时间"(w438) -> ()
                    }
                    frame 3 {
                      n386 = global write "全局 时间2.vi" "CODMn零点核查索引起始时间"(w439) -> ()
                      n387 = global write "全局 时间2.vi" "CODMn跨度核查索引起始时间"(w439) -> ()
                    }
                    frame 4 {
                      n388 = global write "全局 时间2.vi" "CODCr零点核查索引起始时间"(w440) -> ()
                      n389 = global write "全局 时间2.vi" "CODCr跨度核查索引起始时间"(w440) -> ()
                    }
                  }
                }
              }
              frame True {
              }
            }
          }
        }
      }
      event "开机启动": Value Change {
        n390 = event-data() -> ("NewVal"=w463:bool)  [unwired: 1 in, 5 out]
        n391 = case shown="假" w463 {
          frame False {
            n392 = Two Button Dialog(message="是否删除开机启动？" ("消息"), 1:"否" ("F按钮名称（“取消”）"), 2:"是" ("T按钮名称（“确定”）")) -> (T button?=w464:bool)
            n393 = case shown="真" w464 {
              frame False {
              }
              frame True {
                n394 = call <vilib>:"Application Directory.vi"() -> ("Application Directory"=w469:path)
                n395 = call "删除启动项.vi"("启动文件路径"=w469) -> ("删除标记"=w468:bool)  [unwired: 9 in, 1 out]
                n396 = case shown="假" w468 {
                  tunnel: ["删除开机启动失败" ("T按钮名称（“确定”）") "删除开机启动成功" ("T按钮名称（“确定”）")] -> w470
                  frame False {
                  }
                  frame True {
                  }
                }
                n397 = One Button Dialog(message=w470) -> ()  [unwired: 1 in, 1 out]
              }
            }
          }
          frame True {
            n398 = Two Button Dialog(message="是否添加开机启动？" ("消息"), 1:"否" ("F按钮名称（“取消”）"), 2:"是" ("T按钮名称（“确定”）")) -> (T button?=w473:bool)
            n399 = case shown="真" w473 {
              frame False {
              }
              frame True {
                n400 = call <vilib>:"Application Directory.vi"() -> ("Application Directory"=w479:path)
                n401 = call "添加启动项.vi"("启动文件路径"=w479) -> ("添加成功标记"=w478:bool)  [unwired: 9 in, 1 out]
                n402 = case shown="真" w478 {
                  tunnel: ["添加开机启动失败" ("T按钮名称（“确定”）") "添加开机启动成功" ("T按钮名称（“确定”）")] -> w477
                  frame False {
                  }
                  frame True {
                  }
                }
                n403 = One Button Dialog(message=w477) -> ()  [unwired: 1 in, 1 out]
              }
            }
          }
        }
      }
      event "IP", "PORT": Mouse Down {
        n404 = event-data() -> ("CtlRef"=w485:refnum<vi>)  [unwired: 1 in, 7 out]
        n405 = property class="Str"(reference=w485) -> (reference out=w483:refnum<vi>, "Value"=w484:string)  [unwired: 1 in, 1 out]
        n406 = call "IP键盘.vi"("OldNumber"=w484) -> ("NewNumber"=w482:string)
        n407 = property class="Str"(reference=w483, "Val(Sgnl)"=w482) -> ()  [unwired: 1 in, 2 out]
      }
    }
  }
  n408 = case shown="\"Development System\", 默认" w5 {
    tunnel: [T12."Standard" ("状态") T12."Hidden" ("状态")] -> w32
    frame "Development System", Default {
    }
    frame "Run Time System" {
    }
  }
  n409 = Obtain Queue(name (unnamed)="actualwrite" ("名称（未命名）"), element data type=enum16{"打开连接", "发送数据", "读取数据", "数据处理", "关闭连接"}."打开连接" ("枚举")) -> (queue out=w45:refnum<queue>, error out=w44:errorcluster)  [unwired: 3 in, 1 out]
  n410 = Obtain Queue(name (unnamed)="actualread" ("名称（未命名）"), element data type=enum16{"打开连接", "发送数据", "读取数据", "数据处理", "关闭连接"}."打开连接" ("枚举")) -> (queue out=w55:refnum<queue>, error out=w48:errorcluster)  [unwired: 3 in, 1 out]
  n411 = property class="VI"(reference=w42) -> ("Name"=w41:string)  [unwired: 1 in, 2 out]
  n412 = while {
    tunnel: w45 -> [w496]
    tunnel: w44 -> [w495]
    shift-right: [w491] -> _
    shift-left: errorcluster {"status"=FALSE, "code"=0, "source"=""} ("error out") -> [w490]
    stop <- FALSE stop-if-true
    # "写入数据出队列"
    n413 = Dequeue Element(queue=w496, timeout in ms (-1)=30000 ("超时毫秒(-1)"), error in (no error)=w495) -> (queue out=w489:refnum<queue>, element=w493:enum16{"打开连接", "发送数据", "读取数据", "数据处理", "关闭连接"}, timed out?=w492:bool, error out=w488:errorcluster)
    n414 = case shown="错误" w490 {
      tunnel: w493 -> [w498 _]
      tunnel: w492 -> [w500 _]
      tunnel: [w504 w544] -> w491
      tunnel: w490 -> [w503 w548]
      tunnel: w489 -> [w502 w546]
      tunnel: w488 -> [w501 w545]
      frame No Error {
        n415 = case shown="真" w500 {
          tunnel: [w505 enum16{"打开连接", "发送数据", "读取数据", "数据处理", "关闭连接"}."发送数据" ("枚举")] -> w499
          tunnel: w498 -> [w505 _]
          frame False {
          }
          frame True {
          }
        }
        n416 = case shown="\"发送数据\", 默认" w499 {
          tunnel: w500 -> [_ w521 _ _ _]
          tunnel: [w507 w524 _ _ w537] -> w504
          tunnel: w503 -> [w509 w523 _ _ w538]
          tunnel: w502 -> [_ _ _ _ w539]
          tunnel: w501 -> [_ _ _ _ w536]
          frame "打开连接" {
            n417 = global read "断电保存全局.vi" "VISA resource name"() -> (w516:refnum<visa-resource-name>)
            n418 = global read "断电保存全局.vi" "数据发送通道"() -> (w513:enum16{"TCP", "VISA"})
            n419 = global read "断电保存全局.vi" "baud rate"() -> (w515:u32)
            n420 = global read "断电保存全局.vi" "PORT"() -> (w514:string)
            n421 = global read "断电保存全局.vi" "IP"() -> (w512:string)
            n422 = call "VISATCP组合选择发送.vi"("IP"=w512, "数据发送通道"=w513, "命令"="open", "PORT"=w514, "VISA resource name"=w516, "baud rate"=w515, "error in (no error)"=w509) -> ("错误输出"=w507:errorcluster)  [unwired: 5 in, 3 out]
            n423 = Unbundle By Name(w507) -> ("status"=w510:bool)  [unwired: 1 out]
            n424 = Not(x=w510) -> (.not. x?=w508:bool)
            n425 = local write "通信状态"(w508) -> ()
          }
          frame "发送数据", Default {
            n426 = case shown="假" w521 {
              tunnel: [w528 w530] -> w518
              tunnel: w523 -> [w527 w531]
              tunnel: [w527 w531] -> w522
              frame False {
                # "事件触发发送数据"
                n427 = global read "全局1.vi" "发送报文显示"() -> (w528:string)
              }
              frame True {
                # "30秒超时发送心跳包"
                n428 = local read "配置信息"() -> (w534:T4)
                n429 = local write "心跳包"(FALSE ("心跳包")) -> ()
                n430 = Unbundle By Name(w534) -> ("MN"=w533:string, "PW"=w532:string)
                n431 = call "数据编码.vi"("table输入"="心跳包", "MN"=w533, "PW"=w532) -> ("通讯包字符串"=w530:string)  [unwired: 11 in, 1 out]
                n432 = global write "全局1.vi" "发送报文显示"(w530) -> ()
              }
            }
            n433 = global read "断电保存全局.vi" "数据发送通道"() -> (w525:enum16{"TCP", "VISA"})
            n434 = Concatenate Strings("send:" ("字符串"), w518) -> (w517:string)
            n435 = call "VISATCP组合选择发送.vi"("数据发送通道"=w525, "命令"="write", "error in (no error)"=w522, "写入缓冲区"=w518) -> ("错误输出"=w524:errorcluster)  [unwired: 8 in, 3 out]
            n436 = Build Array(w517) -> (w520:string[])
            n437 = call "发送数据记录到文档(子VI).vi"("数组"=w520) -> ()  [unwired: 9 in, 1 out]
            "心跳包" <- w521
          }
          frame "读取数据" {
          }
          frame "数据处理" {
          }
          frame "关闭连接" {
            n438 = global read "断电保存全局.vi" "数据发送通道"() -> (w541:enum16{"TCP", "VISA"})
            n439 = Enqueue Element(queue=w539, element=enum16{"打开连接", "发送数据", "读取数据", "数据处理", "关闭连接"}."打开连接" ("枚举"), error in (no error)=w536) -> ()  [unwired: 1 in, 3 out]
            n440 = call "VISATCP组合选择发送.vi"("数据发送通道"=w541, "命令"="close", "error in (no error)"=w538) -> ("错误输出"=w542:errorcluster)  [unwired: 9 in, 3 out]
            n441 = call <vilib>:"Clear Errors.vi"("error in (no error)"=w542) -> ("error out"=w537:errorcluster)  [unwired: 5 in, 1 out]
          }
        }
      }
      frame Error {
        n442 = Unbundle By Name(w548) -> ("code"=w547:i32)
        n443 = case shown="0, 默认" w547 {
          tunnel: w546 -> [w555 w571 w583]
          tunnel: w545 -> [w554 w570 w582]
          tunnel: [w553 w568 w581] -> w544
          frame 0, Default {
            n444 = Flush Queue(queue=w555, error in (no error)=w554) -> (queue out=w557:refnum<queue>, error out=w558:errorcluster)  [unwired: 1 out]
            n445 = local read "状态信息"() -> (w552:T3)
            n446 = Unbundle By Name(w552) -> ("TCP服务端掉线计数"=w550:i32)
            n447 = Enqueue Element(queue=w557, element=enum16{"打开连接", "发送数据", "读取数据", "数据处理", "关闭连接"}."关闭连接" ("枚举"), error in (no error)=w558) -> (error out=w559:errorcluster)  [unwired: 1 in, 2 out]
            n448 = Increment(x=w550) -> (x+1=w551:i32)
            n449 = Bundle By Name(cluster=w552, "TCP服务端掉线计数"=w551) -> (w549:T3)
            n450 = local write "状态信息"(w549) -> ()
            n451 = call <vilib>:"Clear Errors.vi"("error in (no error)"=w559) -> ("error out"=w553:errorcluster)  [unwired: 5 in, 1 out]
          }
          frame 54, 63 {
            n452 = Flush Queue(queue=w571, error in (no error)=w570) -> (queue out=w573:refnum<queue>, error out=w574:errorcluster)  [unwired: 1 out]
            n453 = local read "状态信息"() -> (w563:T3)
            n454 = Unbundle By Name(w563) -> ("TCP服务端掉线计数"=w567:i32, "TCP掉线时间节点"=w560:string)
            n455 = Enqueue Element(queue=w573, element=enum16{"打开连接", "发送数据", "读取数据", "数据处理", "关闭连接"}."关闭连接" ("枚举"), error in (no error)=w574) -> (error out=w569:errorcluster)  [unwired: 1 in, 2 out]
            n456 = Less Or Equal?(x=w567, y=1) -> (x <= y?=w565:bool)
            n457 = case shown="真" w565 {
              tunnel: [w575 w576] -> w564
              tunnel: w560 -> [w575 _]
              frame False {
              }
              frame True {
                n458 = Get Date/Time In Seconds() -> (seconds since 1Jan1904=w577:timestamp)
                n459 = Format Date/Time String(time format string (%c)="%Y%m%d%H%M%S%3u" ("时间格式字符串(%c)"), seconds (now)=w577) -> (date/time string=w579:string)  [unwired: 1 in]
                n460 = call "格式时间字符串.vi"("字符串"=w579) -> ("连接的字符串"=w576:string)  [unwired: 10 in]
              }
            }
            n461 = Increment(x=w567) -> (x+1=w562:i32)
            n462 = call <vilib>:"Clear Errors.vi"("error in (no error)"=w569) -> ("error out"=w568:errorcluster)  [unwired: 5 in, 1 out]
            n463 = Bundle By Name(cluster=w563, "TCP服务端掉线计数"=w562, "TCP掉线时间节点"=w564) -> (w561:T3)
            n464 = local write "状态信息"(w561) -> ()
          }
          frame 56 {
            n465 = Flush Queue(queue=w583, error in (no error)=w582) -> (error out=w580:errorcluster)  [unwired: 2 out]
            n466 = call <vilib>:"Clear Errors.vi"("error in (no error)"=w580) -> ("error out"=w581:errorcluster)  [unwired: 5 in, 1 out]
          }
        }
      }
    }
  }
  n467 = call <vilib>:"Application Directory.vi"() -> ("Application Directory"=w11:path)
  n468 = Open VI Reference(type specifier VI Refnum (for type only)=refnum<vi> refnum, vi path=w41, options=128 ("选项")) -> (vi reference=w39:refnum<vi>, error out=w37:errorcluster)  [unwired: 3 in]
  n469 = Build Path(base path=w11, name or relative path="data\\tubiao.ico" ("名称或相对路径")) -> (appended path=w21:path)
  n470 = Enqueue Element(queue=w55, element=enum16{"打开连接", "发送数据", "读取数据", "数据处理", "关闭连接"}."打开连接" ("枚举"), error in (no error)=w48) -> (queue out=w51:refnum<queue>, error out=w50:errorcluster)  [unwired: 1 in, 1 out]
  n471 = Obtain Queue(name (unnamed)="datasent" ("名称（未命名）"), element data type=enum16{"实时小时数据", "核查数据日志信息", "其他信息", "反控命令"}."核查数据日志信息") -> (queue out=w2:refnum<queue>, error out=w1:errorcluster)  [unwired: 3 in, 1 out]
  n472 = Current VI's Path() -> (path=w8:path)
  n473 = call-by-ref "?"(reference=w39, error in=w37) -> (reference out=w35:refnum<vi>, error out=w36:errorcluster)  [unwired: 12 in]
  n474 = Build Array(w21) -> (w16:path[])
  n475 = Open VI Reference(vi path=w8) -> (vi reference=w7:refnum<vi>)  [unwired: 5 in, 1 out]
  n476 = Close Reference(reference=w35, error in (no error)=w36) -> ()  [unwired: 1 out]
  n477 = while {
    tunnel: w51 -> [w594]
    tunnel: w50 -> [w593]
    shift-right: [w590] -> _
    shift-left: errorcluster {"status"=FALSE, "code"=0, "source"=""} ("error out") -> [w589]
    tunnel: w2 -> [w585]
    tunnel: w1 -> [w584]
    stop <- FALSE stop-if-true
    # "读取数据出队列处理"
    n478 = Dequeue Element(queue=w594, error in (no error)=w593) -> (queue out=w588:refnum<queue>, element=w591:enum16{"打开连接", "发送数据", "读取数据", "数据处理", "关闭连接"}, error out=w587:errorcluster)  [unwired: 1 in, 1 out]
    n479 = Wait (ms)(milliseconds to wait=u32 1000 ("等待时间（毫秒）")) -> ()  [unwired: 1 out]
    n480 = case shown="无错误" w589 {
      tunnel: w591 -> [w598 _]
      tunnel: [w605 w668] -> w590
      tunnel: w589 -> [w604 w672]
      tunnel: w588 -> [w603 w670]
      tunnel: w587 -> [w602 w669]
      tunnel: w585 -> [w596 _]
      tunnel: w584 -> [w595 _]
      frame No Error {
        n481 = case shown="\"打开连接\", 默认" w598 {
          tunnel: [w612 _ w644 _ w663] -> w605
          tunnel: w604 -> [w611 _ w647 _ w664]
          tunnel: w603 -> [w609 _ w639 _ w661]
          tunnel: w602 -> [w608 _ w638 _ w660]
          tunnel: [w607 _ _ _ _] -> w599
          tunnel: w596 -> [_ _ w630 _ _]
          tunnel: w595 -> [_ _ w629 _ _]
          frame "打开连接", Default {
            n482 = Enqueue Element(queue=w609, element=enum16{"打开连接", "发送数据", "读取数据", "数据处理", "关闭连接"}."读取数据" ("枚举"), error in (no error)=w608) -> ()  [unwired: 1 in, 3 out]
            n483 = global read "断电保存全局.vi" "VISA resource name"() -> (w619:refnum<visa-resource-name>)
            n484 = global read "断电保存全局.vi" "数据发送通道"() -> (w616:enum16{"TCP", "VISA"})
            n485 = global read "断电保存全局.vi" "baud rate"() -> (w618:u32)
            n486 = global read "断电保存全局.vi" "PORT"() -> (w617:string)
            n487 = global read "断电保存全局.vi" "IP"() -> (w615:string)
            n488 = call "VISATCP组合选择发送.vi"("IP"=w615, "数据发送通道"=w616, "命令"="open", "PORT"=w617, "VISA resource name"=w619, "baud rate"=w618, "error in (no error)"=w611) -> ("错误输出"=w612:errorcluster)  [unwired: 5 in, 3 out]
            n489 = Unbundle By Name(w612) -> ("status"=w606:bool, "code"=w607:i32)
            n490 = Not(x=w606) -> (.not. x?=→"通信状态":bool)
            n491 = global write "全局 数据发送重叠.vi" "掉线指示灯"(w606) -> ()
          }
          frame "发送数据" {
          }
          frame "读取数据" {
            n492 = Get Queue Status(queue=w639, error in (no error)=w638) -> (queue out=w635:refnum<queue>, error out=w634:errorcluster, # elements in queue=w637:i32)  [unwired: 1 in, 5 out]
            n493 = global read "断电保存全局.vi" "数据发送通道"() -> (w646:enum16{"TCP", "VISA"})
            n494 = Equal To 0?(x=w637) -> (x = 0?=w636:bool)
            n495 = case shown="真" w636 {
              tunnel: w635 -> [_ w658]
              tunnel: w634 -> [_ w657]
              frame False {
              }
              frame True {
                n496 = Enqueue Element(queue=w658, element=enum16{"打开连接", "发送数据", "读取数据", "数据处理", "关闭连接"}."读取数据" ("枚举"), error in (no error)=w657) -> ()  [unwired: 1 in, 3 out]
              }
            }
            n497 = call "VISATCP组合选择发送.vi"("数据发送通道"=w646, "命令"="read", "error in (no error)"=w647) -> ("读取缓冲区"=w632:string, "错误输出"=w644:errorcluster)  [unwired: 9 in, 2 out]
            n498 = call "读取数据处理 (子VI).vi"("data out"=w632) -> ("命令编码CN"=w640:string, "数据"=w627:string, "时间QN"=w631:string)  [unwired: 8 in, 4 out]
            n499 = Empty String/Path?(string/path=w632) -> (empty?=w633:bool)
            n500 = case shown="假" w633 {
              tunnel: w632 -> [w653 _]
              tunnel: w631 -> [w654 _]
              frame False {
                n501 = global write "全局1.vi" "QN"(w654) -> ()
                n502 = global write "全局1.vi" "数据输出"(w653) -> ()
                n503 = global write "全局1.vi" "读取报文显示"(w653) -> ()
                n504 = call "数据记录.vi"("写入字段"=w653) -> ("连接的字符串"=w655:string)  [unwired: 10 in]
                n505 = Build Array(w655) -> (w656:string[])
                n506 = call "发送数据记录到文档(子VI).vi"("数组"=w656) -> ()  [unwired: 9 in, 1 out]
              }
              frame True {
              }
            }
            n507 = Search/Split String(string=w640, search string/char (-)="CN=" ("搜索字符串/字符(-)")) -> (match + rest of string=w641:string)  [unwired: 1 in, 2 out]
            n508 = String Subset(string=w641, offset (0)=3 ("偏移量(0)")) -> (substring=w625:string)  [unwired: 1 in]
            n509 = Empty String/Path?(string/path=w625) -> (empty?=w628:bool)
            n510 = Not Equal?(x=w625, y="9013") -> (x != y?=w622:bool)
            n511 = Not Equal?(x=w625, y="9014") -> (x != y?=w621:bool)
            n512 = Not(x=w628) -> (.not. x?=w620:bool)
            n513 = Compound Arithmetic op=AND ("复合运算")(w620, w622, w621) -> (w626:bool)
            n514 = case shown="真" w626 {
              tunnel: w630 -> [_ w651]
              tunnel: w629 -> [_ w650]
              tunnel: w627 -> [_ w649]
              tunnel: w625 -> [_ w648]
              frame False {
              }
              frame True {
                n515 = global write "全局1.vi" "命令编码CN"(w648) -> ()
                n516 = global write "全局1.vi" "数据"(w649) -> ()
                n517 = Enqueue Element(queue=w651, element=enum16{"实时小时数据", "核查数据日志信息", "其他信息", "反控命令"}."反控命令", error in (no error)=w650) -> ()  [unwired: 1 in, 3 out]
              }
            }
          }
          frame "数据处理" {
          }
          frame "关闭连接" {
            n518 = global read "断电保存全局.vi" "数据发送通道"() -> (w666:enum16{"TCP", "VISA"})
            n519 = Enqueue Element(queue=w661, element=enum16{"打开连接", "发送数据", "读取数据", "数据处理", "关闭连接"}."打开连接" ("枚举"), error in (no error)=w660) -> ()  [unwired: 1 in, 3 out]
            n520 = call "VISATCP组合选择发送.vi"("数据发送通道"=w666, "命令"="close", "error in (no error)"=w664) -> ("错误输出"=w665:errorcluster)  [unwired: 9 in, 3 out]
            n521 = call <vilib>:"Clear Errors.vi"("error in (no error)"=w665) -> ("error out"=w663:errorcluster)  [unwired: 5 in, 1 out]
          }
        }
        n522 = local read "状态信息"() -> (w601:T3)
        n523 = Bundle By Name(cluster=w601, "TCP服务端掉线计数"=0, "1st Error to Convert"=w599, "步骤"=w598) -> (→"状态信息":T3)
      }
      frame Error {
        n524 = Unbundle By Name(w672) -> ("code"=w671:i32)
        n525 = case shown="54, 63" w671 {
          tunnel: w670 -> [w679 w695 w706]
          tunnel: w669 -> [w678 w694 w705]
          tunnel: [w677 w692 w704] -> w668
          frame 0, Default {
            n526 = Flush Queue(queue=w679, error in (no error)=w678) -> (queue out=w681:refnum<queue>, error out=w682:errorcluster)  [unwired: 1 out]
            n527 = local read "状态信息"() -> (w676:T3)
            n528 = Enqueue Element(queue=w681, element=enum16{"打开连接", "发送数据", "读取数据", "数据处理", "关闭连接"}."关闭连接" ("枚举"), error in (no error)=w682) -> (error out=w683:errorcluster)  [unwired: 1 in, 2 out]
            n529 = Unbundle By Name(w676) -> ("TCP服务端掉线计数"=w674:i32)
            n530 = Increment(x=w674) -> (x+1=w675:i32)
            n531 = Bundle By Name(cluster=w676, "TCP服务端掉线计数"=w675) -> (w673:T3)
            n532 = local write "状态信息"(w673) -> ()
            n533 = call <vilib>:"Clear Errors.vi"("error in (no error)"=w683) -> ("error out"=w677:errorcluster)  [unwired: 5 in, 1 out]
          }
          frame 54, 63 {
            n534 = Flush Queue(queue=w695, error in (no error)=w694) -> (queue out=w697:refnum<queue>, error out=w698:errorcluster)  [unwired: 1 out]
            n535 = local read "状态信息"() -> (w687:T3)
            n536 = Unbundle By Name(w687) -> ("TCP服务端掉线计数"=w691:i32, "TCP掉线时间节点"=w684:string)
            n537 = Enqueue Element(queue=w697, element=enum16{"打开连接", "发送数据", "读取数据", "数据处理", "关闭连接"}."关闭连接" ("枚举"), error in (no error)=w698) -> (error out=w693:errorcluster)  [unwired: 1 in, 2 out]
            n538 = Less Or Equal?(x=w691, y=1) -> (x <= y?=w689:bool)
            n539 = Increment(x=w691) -> (x+1=w686:i32)
            n540 = case shown="真" w689 {
              tunnel: [w699 w700] -> w688
              tunnel: w684 -> [w699 _]
              frame False {
              }
              frame True {
                n541 = Get Date/Time In Seconds() -> (seconds since 1Jan1904=w701:timestamp)
                n542 = Format Date/Time String(time format string (%c)="%Y%m%d%H%M%S%3u" ("时间格式字符串(%c)"), seconds (now)=w701) -> (date/time string=w703:string)  [unwired: 1 in]
                n543 = call "格式时间字符串.vi"("字符串"=w703) -> ("连接的字符串"=w700:string)  [unwired: 10 in]
              }
            }
            n544 = call <vilib>:"Clear Errors.vi"("error in (no error)"=w693) -> ("error out"=w692:errorcluster)  [unwired: 5 in, 1 out]
            n545 = Bundle By Name(cluster=w687, "TCP服务端掉线计数"=w686, "TCP掉线时间节点"=w688) -> (w685:T3)
            n546 = local write "状态信息"(w685) -> ()
          }
          frame 56 {
            n547 = Flush Queue(queue=w706, error in (no error)=w705) -> (queue out=w708:refnum<queue>, error out=w709:errorcluster)  [unwired: 1 out]
            n548 = Enqueue Element(queue=w708, element=enum16{"打开连接", "发送数据", "读取数据", "数据处理", "关闭连接"}."读取数据" ("枚举"), error in (no error)=w709) -> (error out=w710:errorcluster)  [unwired: 1 in, 2 out]
            n549 = call <vilib>:"Clear Errors.vi"("error in (no error)"=w710) -> ("error out"=w704:errorcluster)  [unwired: 5 in, 1 out]
          }
        }
      }
    }
  }
  n550 = invoke class="VI" method="FP.Open"(reference=w7, "Activate"=TRUE ("激活？"), "State"=w32) -> (error out=w6:errorcluster)  [unwired: 2 in, 4 out]
  n551 = call <vilib>:"Constructor.vi"("error in"=w6, "IconFilePathList"=w16) -> ("error out"=w20:errorcluster, "NotifyIcon"=w12:refnum<class "NotifyIcon.lvclass">)  [unwired: 8 in]
  n552 = for {
    shift-right: [w715] -> w34
    shift-left: w20 -> [w716]
    tunnel: string[] ["Open", "-", "Exit"] -> [w714] mode=indexing
    tunnel: w13 -> [w713] mode=indexing
    shift-right: [w711] -> w33
    shift-left: w12 -> [w712]
    # "2."
    n553 = call <vilib>:"InsertMenuItem.vi"("error in"=w716, "ItemTag"=w713, "ItemName"=w714, "NotifyIcon in"=w712) -> ("error out"=w715:errorcluster, "NotifyIcon out"=w711:refnum<class "NotifyIcon.lvclass">)  [unwired: 6 in]
  }
  n554 = Index Array(array=w13) -> (element=w14:string)  [unwired: 1 in]
  n555 = property class="NotifyIcon"(reference=w33, error in=w34, "Public:Visible"=TRUE ("Visible"), "Public:DefaultMenuItem"=w14, "Public:TipText"="平台数据传输系统" ("TipText")) -> (reference out=w28:refnum<class "NotifyIcon.lvclass">, error out=w19:errorcluster, "Public:SelectedItemEvent"=w18:refnum<user-event>)
  n556 = register-events(error in=w19, w18) -> (reference out=w29:refnum<event-registration>, error out=w30:errorcluster)  [unwired: 1 in]
  n557 = while {
    shift-right: [w720] -> w26
    shift-left: w30 -> [w719]
    shift-right: [w721] -> w23
    shift-left: w28 -> [w722]
    shift-right: [w718] -> w24
    shift-left: w29 -> [w723]
    tunnel: [w717] -> _
    stop <- w717 stop-if-true
    n558 = case shown="无错误" w719 {
      selector: w719 -> [w725 w759]
      tunnel: w723 -> [w730 w754]
      tunnel: w722 -> [w729 w755]
      tunnel: [w728 w755] -> w721
      tunnel: [w727 w757] -> w720
      tunnel: [w726 FALSE ("Discard?")] -> w717
      tunnel: [w724 w754] -> w718
      frame No Error {
        n559 = event shown="[0] <Public:SelectedItemEvent>: 用户事件" {
          selector: w730 -> [_ _ _]
          dyn-events: [_ _ _] -> w724
          timeout: _ -> [_ _ _]
          tunnel: w725 -> [w733 w743 w752]
          tunnel: [w733 w743 w751] -> w727
          tunnel: [w732 TRUE FALSE ("Discard?")] -> w726
          tunnel: w729 -> [w731 w741 w753]
          tunnel: [w731 w741 w750] -> w728
          event User Event {
            # "5."
            n560 = event-data() -> ("ItemTag"=w734:string)  [unwired: 1 in]
            n561 = case shown="默认" w734 {
              tunnel: [FALSE TRUE] -> w732
              frame Default {
                n562 = Current VI's Path() -> (path=w735:path)
                n563 = Open VI Reference(vi path=w735) -> (vi reference=w736:refnum<vi>)  [unwired: 5 in, 1 out]
                n564 = invoke class="VI" method="FP.Open"(reference=w736, "Activate"=TRUE ("激活？")) -> ()  [unwired: 3 in, 5 out]
              }
              frame "EXIT" {
              }
            }
          }
          event "停止输入": Value Change {
            # "5."
            n565 = event-data() -> ()  [unwired: 1 in, 6 out]
            n566 = Stop(stop? (T)=TRUE ("可见")) -> ()
          }
          event Panel Close? {
            # "4."
            n567 = event-data() -> ("VIRef"=w746:refnum<vi>)  [unwired: 1 in, 3 out]
            n568 = invoke class="VI" method="FP.Open"(reference=w746, "State"=T12."Hidden" ("状态")) -> ()  [unwired: 3 in, 5 out]
            n569 = call <vilib>:"ShowBalloonTip.vi"("Balloon Icon"=BalloonIcon."Information", "error in"=w752, "Text"="欢迎使用平台数据传输系统", "NotifyIcon in"=w753) -> ("error out"=w751:errorcluster, "NotifyIcon out"=w750:refnum<class "NotifyIcon.lvclass">)  [unwired: 6 in]
            n570 = event-data("Discard?"=TRUE ("放弃？")) -> ()  [unwired: 1 in, 1 out]
          }
        }
      }
      frame Error {
        n571 = call <vilib>:"Simple Error Handler.vi"("error in (no error)"=w759) -> ("error out"=w758:errorcluster)  [unwired: 4 in, 4 out]
        n572 = call <vilib>:"Clear Errors.vi"("error in (no error)"=w758) -> ("error out"=w757:errorcluster)  [unwired: 5 in, 1 out]
      }
    }
  }
  n573 = Unregister For Events(event registration refnum=w24, error in=w26) -> (error out=w27:errorcluster)
  n574 = call <vilib>:"Destructor.vi"("error in"=w27, "NotifyIcon"=w23) -> ("error out"=w22:errorcluster)  [unwired: 9 in]
  n575 = call <vilib>:"Simple Error Handler.vi"("error in (no error)"=w22) -> ("error out"=→"错误输出":errorcluster)  [unwired: 4 in, 4 out]
  n576 = case shown="\"Embedded LabVIEW\"" w5 {
    tunnel: w22 -> [_ _ _ _ _ _ _]
    frame "invalid app kind", Default {
    }
    frame "Development System" {
      n577 = Stop(stop? (T)=TRUE ("可见")) -> ()
    }
    frame "Run Time System" {
      n578 = Quit LabVIEW(quit? (T)=TRUE ("退出？(T)")) -> ()
    }
    frame "Student Edition" {
    }
    frame "Embedded LabVIEW" {
    }
    frame "Evaluation" {
    }
    frame "Custom" {
    }
  }
